vi "UHR-Fleezers Control (fpga) - 10.8b.vi"() -> ()   [LabVIEW 2014]
doc: "UHR-Fleezers Instrument Control Code (fpga)"
uses:
  <vilib>/eio/EIONode/EIONode.xnode
  <vilib>/eio/EIOMethodNode/EIOMethodNode.xnode
  <vilib>/rvi/DataTransferAndStorage/Container/XNode/niFpgaContainer.xnode
  <vilib>/Platform/TimedLoop/XDataNode/XDataNode.xnode
  <vilib>/Platform/TimedLoop/XDataNode/nitl_modes.ctl
  <vilib>/Platform/TimedLoop/XDataNode/XDNodeRunTimeDep.lvlib
  <vilib>/Platform/TimedLoop/XDataNode/wakeup.ctl
  <vilib>/Platform/TimedLoop/XDataNode/timing_clust.ctl
  <vilib>/addons/control/pid/fpga.llb/XNode/niFpgaPID.xnode
  <vilib>/rvi/eio/common/nirviEmuTemplateMethod_errors.vi
  <vilib>/rvi/interface/RandomDataEmulation/nirviRandomDataFpgaReadWriteTemplate.vi
panel:
  in  "Connector0/AO6":i16
  in  "Tab Control":T1(tab)=enum."Force FB"
  in  "Trap Pos to FIFO":bool
  in  "AI1 Sets to FIFO":T2={"Set 1"=TRUE, "Set 2"=TRUE, "Set 3"=FALSE}
  in  "N of AI1 Int Acq Sets":i16=2 min=1 max=3 step=1
  out "AI Late Counter":u16
  in  "ai count":u32=400
  out "AI late?":bool
  in  "+ phase":bool
  in  "Phase count adjustment":i16
  out "Relative phase":i16
  in  "AI to FIFO":bool
  out "BD1 Frequency Out 1":u64
  out "BD1 Frequency Out 2":u64
  out "Trap Pos FIFO Timeout":u16
  out "Trap AI FIFO Timeout":u16
  in  "Trap FIFO Set Timeout":i32
  in  "Tab Control 2":T3(tab)
  out "Wiggling 2":bool
  in  "Abort wiggle 2":bool
  in  "Wiggle amp 2":u64
  in  "Wiggle freq 2 (Hz)":fxp<+/-,16,16>
  in  "Wiggle trap 2":bool
  out "Wiggling 1":bool
  in  "Abort wiggle 1":bool
  in  "Wiggle trap 1":bool
  in  "Wiggle amp 1":u64
  in  "Wiggle freq 1 (Hz)":fxp<+/-,16,16>
  in  "Swap F1 and F2":bool
  in  "Freq or Amp switch first":bool=TRUE
  in  "Cont. Scan":bool
  in  "Abort scan":bool
  in  "Cycles per step":u64
  in  "Scan BD":bool
  in  "Number of scans":u16
  in  "Scan steps":u64
  in  "Scan freq.  increment":i64
  out "Scanning":bool
  in  "Start scan":bool
  in  "OSK Bd 1":bool
  in  "Reset Bd 1":bool
  in  "RD":bool
  in  "PMODE":bool
  in  "OSK Bd 2":bool
  in  "Reset Bd 2":bool
  in  "Direct RF Box \nCommunication":bool
  in  "Data BD 2":u8 format="%08b"
  in  "Data BD 1":u8 format="%08b"
  in  "Address":u8 format="%02x"
  in  "Update Data":bool
  in  "FPGA Controls\n RF Box":bool
  in  "Number Interlace Cycles":u8=2 min=1 max=3
  in  "Interlace Off Parameters":u8=1 min=1 max=3
  in  "Interlace ON/OFF":bool
  out "DIO Relative phase":i16
  in  "Phase count adjustment (DIO)":i16
  in  "+ phase (DIO)":bool
  out "DIO Late Counter":u16
  out "DIO Late?":bool
  in  "DIO count 1 (ticks)":u32=400
  in  "DIO count 2 (ticks)":u32=400
  in  "DIO count 3 (ticks)":u32=400
  out "AI2 Y Sum Set 2":i16
  out "AI2 Y Sum Set 1":i16
  in  "FB Gains Set 1":T4={"proportional gain (Kc)"=10, "integral gain (Kc*Ts/Ti)"=5, "derivative gain (Kc*Td/Ts)"=0}
  in  "FB Setpoint Set 1":i16 min=0 step=1
  in  "FB Reset Set 1":bool
  in  "FB On/Off Set 1":bool
  in  "FB Reset Set 2":bool
  in  "FB On/Off Set 2":bool
  in  "FB Setpoint Set 2":i16 min=0 step=1
  in  "FB Gains Set 2":T4={"proportional gain (Kc)"=10, "integral gain (Kc*Ts/Ti)"=5, "derivative gain (Kc*Td/Ts)"=0}
  in  "FB output range 2":cluster{"output high":i16, "output low":i16}={"output high"=3000, "output low"=0}
  in  "FB output range 1":cluster{"output high":i16, "output low":i16}={"output high"=3000, "output low"=0}
  out "Scan I":u64
  in  "Amp switch delay":u16=5
  in  "Freq switch delay":u16
  in  "BD 2 Amplitude 1":u16
  in  "BD 1 Amplitude 1":u16
  in  "BD 2 Frequency 1":u64
  in  "BD 1 Frequency 1":u64
  in  "BD 2 Amplitude 2":u16
  in  "BD 1 Amplitude 2":u16
  in  "BD 2 Frequency 2":u64
  in  "BD 1 Frequency 2":u64
  in  "BD 2 Amplitude 3":u16
  in  "BD 1 Amplitude 3":u16
  in  "BD 2 Frequency 3":u64
  in  "BD 1 Frequency 3":u64
  in  "Negate Diff?":bool
  in  "Diff FB Measurement?":bool
  in  "FB Trig Integrate":u32=1
  out "TTrig?":bool
  in  "TTrig Negate Pos":bool=TRUE
  out "Trap Pos FB Int Signal":fxp<+/-,24,9> format="%.18g"
  out "Trap Pos FB Int-Norm Signal":fxp<+/-,16,1> format="%.16g"
  in  "FPGA TTrig Thresh":i64
  in  "FPGA Trap Trig":bool
  out "Trap Pos FB Action":i64
  in  "Trap Pos. FB Offset Factor":i64
  in  "Trap Pos. FB Mult Factor":i64=2
  in  "Trap Pos. FB Range":T5={"output high"=0.999969482421875, "output low"=-1.0}
  in  "Trap Pos. FB Gains":T6={"proportional gain (Kc)"=0.0, "integral gain (Kc*Ts/Ti)"=10.0, "derivative gain (Kc*Td/Ts)"=0.0} {"proportional gain (Kc)" format="%.11g"; "integral gain (Kc*Ts/Ti)" format="%.11g"; "derivative gain (Kc*Td/Ts)" format="%.11g"}
  in  "Trap Pos. FB Reset":bool
  in  "Trap Pos FB Monitor T1 or T2":bool
  in  "AI1 X Scale":u16
  in  "Trap Pos FB Int Count":u16=100
  in  "Trap Pos FB Negate Action":bool
  out "AI1 X Set 2":fxp<+/-,16,1>
  out "AI1 X Set 1":fxp<+/-,16,1>
  in  "Trap Pos. FB SP":fxp<+/-,16,1>
  in  "Force feedback":bool
  out "TTrig Sig":i64
  out "TTrig Fin Thresh":i64
  out "Numeric":i32
  out "AO2 2":i16
  out "AO1 2":i16
  in  "1D or 2D Scan?":bool
  in  "Abort scan (MCL)":bool
  in  "MCL Scan Axis":bool
  in  "Cont. Scan (MCL)":bool
  out "Scan I (MCL)":u64
  in  "Number of scans (MCL)":u16
  out "Scanning MCL":bool
  in  "Scan steps (MCL)":u64
  in  "Cycles per step (MCL)":u64
  in  "Scan freq.  increment (MCL)":i16
  in  "Start scan (MCL)":bool
  in  "AO2":i16
  in  "AO1":i16
  out "MCL Late Counter":u16
  out "MCL Late?":bool
  in  "MCL count":u32=800
  out "MCL Relative Phase":i16
  in  "Phase count adjustment (MCL)":i16
  in  "+ phase (MCL)":bool
  in  "APD Gate Operating Mode":u8 max=2 step=1
  in  "Invert APD Gate":bool
  in  "APD Gate OFF Count":u32=100
  in  "APD Gate ON Count":u32=300
  out "APD 1 Gate Late Counter":u16
  out "APD 1 Gate Late?":bool
  out "APD 1 Gate Relative Phase":i16
  in  "Phase count adjustment (APD 1 Gate)":i16
  in  "+ phase (APD 1 Gate)":bool
  out "APD 2 Counts 0":u32
  out "APD 2 Counts 1":u32
  out "APD 1 Counts 0":u32
  out "APD 1 Counts 1":u32
  out "APD 1 out state":bool
  in  "APD 2 AO scale factor":i16=1
  in  "APD 1 AO scale factor":i16=1
  in  "APD to FIFO":bool
  in  "APD Acq Rate Count":u32=20000000
  out "APD Acq Late Counter":u16
  out "APD Acq Late?":bool
  out "APD Acq Relative Phase":i16
  in  "Phase Count Adjustment (APD Acq)":i16
  in  "+ phase (APD Acq)":bool
  in  "Phase count adjustment (APD 2 Gate)":i16
  out "APD 2 Gate Late Counter":u16
  out "APD 2 Gate Late?":bool
  out "APD 2 Gate Relative Phase":i16
  in  "+ phase (APD 2 Gate)":bool
  out "APD 2 out state":bool
  out "APD 1 Int Gate":bool
  out "APD 2 Int Gate":bool
  in  "Green Filter Flipper":bool
  out "Green FB Signals":T7
  in  "Green FB Count":u32=1200
  out "Green Late Counter":u16
  out "Green FB Late?":bool
  out "Green FB Relative Phase":i16
  in  "Phase count adjustment (Green FB)":i16=10
  in  "+ phase (Green FB)":bool
  out "Green FB Sum":i16
  in  "Green int current ON count adj":u32=150
  in  "Current Out":u16=30000
  in  "Green FB On/Off":bool
  in  "Green FB Setpoint":i16=250 min=0 step=1
  in  "Green FB Gains":T4={"proportional gain (Kc)"=10, "integral gain (Kc*Ts/Ti)"=5, "derivative gain (Kc*Td/Ts)"=0}
  in  "Green FB Reset":bool
  in  "Operating Mode 2":u8=2 max=2 step=1
  in  "Invert GI 2":bool
  in  "Green interlace OFF count 2":u32=900
  in  "Green interlace ON count 2":u32=300
  out "GI Late Counter 2":u16
  out "GI Late? 2":bool
  out "GI Relative phase 2":i16
  in  "Phase count adjustment (GI) 2":i16=20
  in  "+ phase (GI) 2":bool
  in  "Green interlace OFF count":u32=100
  out "GI Relative phase":i16
  in  "Phase count adjustment (GI)":i16
  in  "+ phase (GI)":bool
  in  "Green interlace ON count":u32=300
  out "GI Late Counter":u16
  in  "Invert GI":bool
  in  "Operating Mode":u8 max=2 step=1
  in  "RI Current Out":u16
  in  "RI operating mode 2":u8
  in  "Red operating mode":u8
  in  "Chassis2/Mod4/AO1":u16
  # "Only one of these can be on\nat a time:"
  # "Raster Scan AOD"
  # "1 (X)"
  # "2 (Y)"
  # "IR Intensity Feedback (RF BD 1)"
  # "FB Triggering Excitation Laser"
  # "AO1 (Y)"
  # "2D"
  # "1D"
  # "AO2 (X)"
  # "APD AO for aligning"
  # "Detection Loop"
  # "Green fluorescent laser digital gate interlacing loop"
  # "0 Forced ON\n1 Forced OFF\n2 Interlacing"
  # "Red fluorescent laser digital gate interlacing loop"
  # "0 Forced ON\n1 Forced OFF\n2 Interlacing"
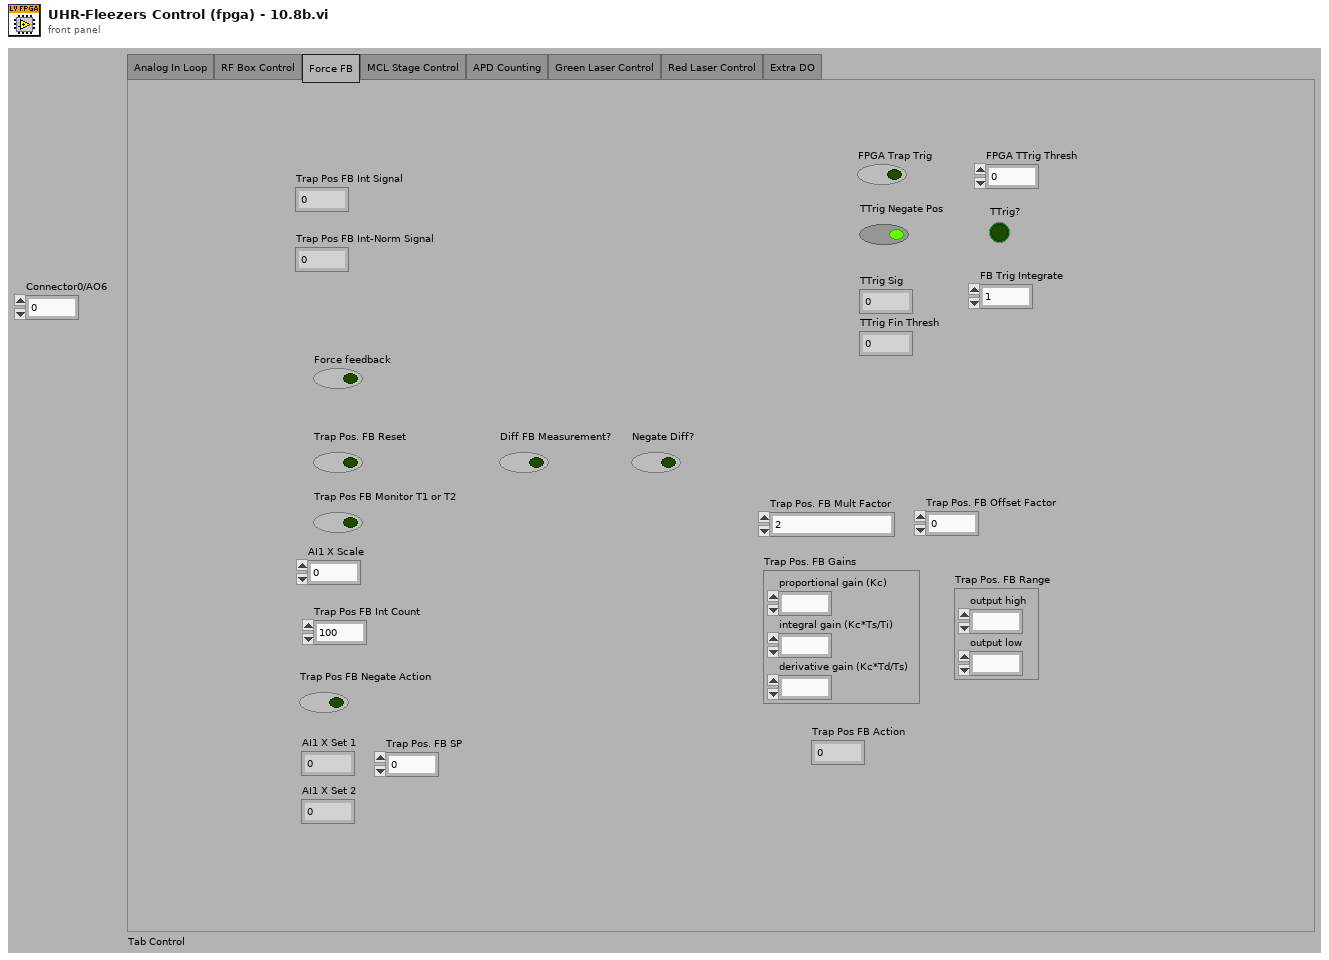
[diagram p1: front panel]
types:
  T1 = enum32{"Analog In Loop", "RF Box Control", "Force FB", "MCL Stage Control", "APD Counting", "Green Laser Control", "Red Laser Control", "Extra DO"}
  T2 = cluster{"Set 1":bool, "Set 2":bool, "Set 3":bool}
  T3 = enum32{"Controls", "Interlacing Frequency and Amplitude Values"}
  T4 = cluster{"proportional gain (Kc)":i16, "integral gain (Kc*Ts/Ti)":i16, "derivative gain (Kc*Td/Ts)":i16}
  T5 = cluster{"output high":fxp<+/-,16,1>, "output low":fxp<+/-,16,1>}
  T6 = cluster{"proportional gain (Kc)":fxp<+/-,16,8>, "integral gain (Kc*Ts/Ti)":fxp<+/-,16,8>, "derivative gain (Kc*Td/Ts)":fxp<+/-,16,8>}
  T7 = cluster{"Green FB Ch 0":i16, "Green FB Ch 1":i16, "Green FB Ch 2":i16}
  T8 = typedef "XDNodeRunTimeDep.lvlib/timing_clust.ctl" = cluster{"Expected End [f-1]":u64, "Actual End [f-1]":u64, "Finished Late? [f-1]":bool, "Expected End [i-1]":u64, "Actual End [i-1]":u64, "Finished Late? [i-1]":bool, "Expected Start [i]":u64, "Actual Start [i]":u64, "Expected Start [f]":u64, "Actual Start [f]":u64, "Source Name":string, "Structure Name":string, "Period":i64, "Deadline":i64, "Offset":i64, "Start":i64, "Priority":i32, "Timeout":i32, "Mode":T9, "Wakeup Reason":T10, "Error":errorcluster, "Source Type":string, "Secondary Source Type":string, "Global End Time":u64, "Global Start Time":u64, "Frame Duration":u64, "Iteration Duration":u64, "Assigned CPU":i32, "I/O Scan Engine Mode":u32}
  T9 = typedef "XDNodeRunTimeDep.lvlib/nitl_modes.ctl" = enum32{"No Change", "Process missed periods, maintain original phase", "Discard missed periods, maintain original phase", "Process missed periods, ignore original phase", "Discard missed periods, ignore original phase"}
  T10 = typedef "XDNodeRunTimeDep.lvlib/wakeup.ctl" = enum32{"Normal", "Aborted", "Asynchronous wakeup", "Timing source error", "Timed loop error", "Timeout"}
  T11 = cluster{"Chassis2/Mod1/AI0":void, "Chassis2/Mod1/AI1":void, "Chassis2/Mod1/AI2":void}
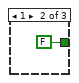
[diagram p2: hidden frame]
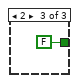
[diagram p3: hidden frame]
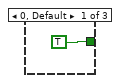
[diagram p4: hidden frame]
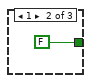
[diagram p5: hidden frame]
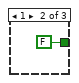
[diagram p6: hidden frame]
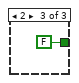
[diagram p7: hidden frame]
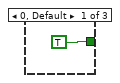
[diagram p9: hidden frame]
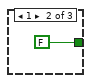
[diagram p10: hidden frame]
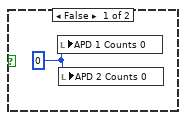
[diagram p11: hidden frame]
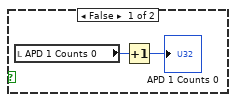
[diagram p14: hidden frame]
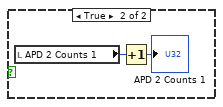
[diagram p16: hidden frame]
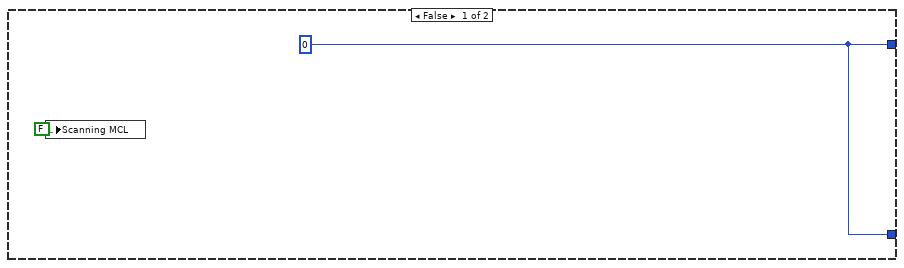
[diagram p17: hidden frame]
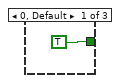
[diagram p18: hidden frame]
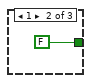
[diagram p19: hidden frame]
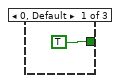
[diagram p20: hidden frame]
diagram:
  w1 = u16 0
  w4 = FALSE
  w2 = FALSE
  # "The APD Int Gate is here so the FPGA will do the integration only when the APD gate is \"ON\" (though we will leave the APD continuously ON now). This was added because the actual APD gating (via the hardware) was giving false signals. -KW"
  # "timing array current index"
  # "timing array"
  # "timing counter (phase adjusted here)"
  # "late counter"
  n1 = flat-sequence "FPGA initialization to do before running any of the loops" {
    tunnel: [u32 0 ("DIO count 3 (ticks)")] -> w3
    tunnel: [w10] -> _
    frame #0 {
      # "Start up expansion chassis early\nto avoid delays later"
      # "This pin controls udclk on the RF boards.\nWhen initially configuring the boards, this pin needs to be\nconfigured as a high impedance input.  Later it will be switched\nto an output."
      # "Initial setting of DIO data and \naddress to low (before reset).  \nThis needs to happen before the other\ncontrol method loops execute."
      n2 = xnode "FPGA I/O Node"("Chassis2/Mod4/AO0"=u16 0) -> ("Chassis2/Mod1/AI0"=w10)  [unwired: 2 in, 2 out]
      n3 = xnode "FPGA I/O Method Node"("Enable"=FALSE) -> ()  [unwired: 1 in, 1 out]
      n4 = xnode "FPGA I/O Node"("Connector1/DIO0"=FALSE, "Connector1/DIO1"=FALSE, "Connector1/DIO2"=FALSE, "Connector1/DIO3"=FALSE, "Connector1/DIO4"=FALSE, "Connector1/DIO5"=FALSE, "Connector1/DIO6"=FALSE, "Connector1/DIO7"=FALSE, "Connector1/DIO8"=FALSE, "Connector1/DIO9"=FALSE, "Connector1/DIO10"=FALSE, "Connector1/DIO11"=FALSE, "Connector1/DIO12"=FALSE, "Connector1/DIO13"=FALSE, "Connector1/DIO15"=FALSE, "Connector1/DIO20"=FALSE, "Connector1/DIO21"=FALSE, "Connector1/DIO22"=FALSE, "Connector1/DIO23"=FALSE, "Connector1/DIO24"=FALSE, "Connector1/DIO25"=FALSE, "Connector1/DIO26"=FALSE, "Connector1/DIO27"=FALSE, "Connector1/DIO14"=FALSE) -> ()  [unwired: 24 in, 24 out]
    }
  }
  n5 = local read "AO1"() -> (w8:i16)
  n6 = local read "AO2"() -> (w7:i16)
  n7 = node-c288() -> (w6:T8)  [unwired: 1 in]
  n8 = while "APD 1 Counter" {
    tunnel: w3 -> [_]
    stop <- FALSE stop-if-true
    n9 = flat-sequence {
      frame #0 {
        n10 = xnode "FPGA I/O Method Node"("FPGA I/O In"=refnum<k21> "Connector0/DIO0" ("APD 1 DO"), "Timeout"=-1) -> ()  [unwired: 2 out]
      }
      frame #1 {
        n11 = local read "APD 1 Int Gate"() -> (w41:bool)
        n12 = case shown="True" w41 {
          frame False {
          }
          frame True {
            n13 = local read "APD 1 out state"() -> (w42:bool)
            n14 = case shown="True" w42 {
              frame False {
                n15 = local read "APD 1 Counts 0"() -> (w44:u32)
                n16 = Increment(x=w44) -> (x+1=→"APD 1 Counts 0":u32)
              }
              frame True {
                n17 = local read "APD 1 Counts 1"() -> (w46:u32)
                n18 = Increment(x=w46) -> (x+1=→"APD 1 Counts 1":u32)
              }
            }
          }
        }
      }
    }
  }
  n19 = while "APD 2 Counter" {
    tunnel: w3 -> [_]
    stop <- FALSE stop-if-true
    n20 = flat-sequence {
      frame #0 {
        n21 = xnode "FPGA I/O Method Node"("FPGA I/O In"=refnum<k21> "Connector0/DIO1" ("APD 2 DO"), "Timeout"=-1) -> ()  [unwired: 2 out]
      }
      frame #1 {
        n22 = local read "APD 2 Int Gate"() -> (w50:bool)
        n23 = case shown="True" w50 {
          frame False {
          }
          frame True {
            n24 = local read "APD 2 out state"() -> (w51:bool)
            n25 = case shown="False" w51 {
              frame False {
                n26 = local read "APD 2 Counts 0"() -> (w53:u32)
                n27 = Increment(x=w53) -> (x+1=→"APD 2 Counts 0":u32)
              }
              frame True {
                n28 = local read "APD 2 Counts 1"() -> (w55:u32)
                n29 = Increment(x=w55) -> (x+1=→"APD 2 Counts 1":u32)
              }
            }
          }
        }
      }
    }
  }
  n30 = while "APD 2 Gating" {
    shift-right: [w59] -> _
    shift-left: w3 -> [w64]
    shift-right: [w58] -> _
    shift-left: w4 -> [w56]
    stop <- FALSE stop-if-true
    n31 = flat-sequence {
      tunnel: w64 -> [w67]
      tunnel: [w68] -> w62
      tunnel: [w67] -> w60
      tunnel: [w66] -> w57
      tunnel: w56 -> [w66]
      tunnel: [w71] -> w63
      tunnel: w62 -> [w71]
      tunnel: [w70] -> w61
      tunnel: w60 -> [w70]
      tunnel: w57 -> [w69]
      tunnel: [w89] -> w59
      tunnel: w63 -> [w100]
      tunnel: w61 -> [w98]
      tunnel: [w93] -> w58
      frame #0 {
        n32 = call "Loop Timer8"("Count(Ticks)"=w67) -> ("Tick Count(Ticks)"=w68:u32)
      }
      frame #1 {
        # "(need 4 channels/APD)"
        n33 = xnode "FPGA I/O Node"("Connector0/DIO8"=w69, "Connector0/DIO9"=w69, "Connector0/DIO10"=w69, "Connector0/DIO11"=w69) -> ()  [unwired: 4 in, 4 out]
        "APD 2 Int Gate" <- w69
      }
      frame #2 {
        n34 = local read "APD Gate ON Count"() -> (w82:u32)
        n35 = local read "APD Gate OFF Count"() -> (w81:u32)
        n36 = feedback #1(TRUE) -> (w95:bool)
        n37 = feedback-in #2(w100) -> ()
        n38 = feedback #2(w100) -> (w83:u32)
        n39 = Not(x=w95) -> (.not. x?=w92:bool)
        n40 = feedback-in #1(w92) -> ()
        n41 = Subtract(x=w100, y=w83) -> (x-y=w99:u32)
        n42 = Select(t=w82, s=w92, f=w81) -> (s? t:f=w97:u32)
        n43 = Subtract(x=w99, y=w98) -> (x-y=w74:u32)
        n44 = Subtract(x=w97, y=w74) -> (x-y=w88:u32)
        n45 = Number To Boolean Array(number=w74) -> (Boolean array=w73:bool[])
        n46 = Or Array Elements(Boolean array=w73) -> (logical OR=w72:bool)
        "APD 2 Gate Late?" <- w72
        n47 = Boolean To (0,1)(Boolean="+ phase (APD 2 Gate)") -> (0, 1=w86:i16)
        n48 = Multiply(x=w86, y="Phase count adjustment (APD 2 Gate)") -> (x*y=w84:i16)
        n49 = Boolean To (0,1)(Boolean=w72) -> (0, 1=w79:i16)
        n50 = Add(x=w88, y=w84) -> (x+y=w89:u32)
        n51 = To Unsigned Word Integer(number=w79) -> (unsigned 16bit integer=w76:u16)
        n52 = feedback #3(i16 0) -> (w91:i16)
        n53 = Subtract(x=w91, y=w84) -> (x-y=w90:i16)
        "APD 2 Gate Relative Phase" <- w90
        n54 = feedback-in #3(w90) -> ()
        n55 = feedback #4(u16 0) -> (w77:u16)
        n56 = Add(x=w76, y=w77) -> (x+y=w75:u16)
        "APD 2 Gate Late Counter" <- w75
        n57 = feedback-in #4(w75) -> ()
        n58 = local read "APD Gate Operating Mode"() -> (w80:u8)
        n59 = case shown="2" w80 {
          tunnel: [TRUE FALSE w106] -> w93
          tunnel: w95 -> [_ _ w104]
          frame 0, Default {
          }
          frame 1 {
          }
          frame 2 {
            n60 = local read "Invert APD Gate"() -> (w103:bool)
            n61 = Not(x=w104) -> (.not. x?=w105:bool)
            n62 = Select(t=w105, s=w103, f=w104) -> (s? t:f=w106:bool)
          }
        }
      }
    }
  }
  n63 = while "APD 1 Gating" {
    shift-right: [w110] -> _
    shift-left: w3 -> [w115]
    shift-right: [w109] -> _
    shift-left: w4 -> [w107]
    stop <- FALSE stop-if-true
    n64 = flat-sequence {
      tunnel: w115 -> [w118]
      tunnel: [w119] -> w113
      tunnel: [w118] -> w111
      tunnel: [w117] -> w108
      tunnel: w107 -> [w117]
      tunnel: [w122] -> w114
      tunnel: w113 -> [w122]
      tunnel: [w121] -> w112
      tunnel: w111 -> [w121]
      tunnel: w108 -> [w120]
      tunnel: [w136] -> w110
      tunnel: w114 -> [w151]
      tunnel: w112 -> [w148]
      tunnel: [w140] -> w109
      frame #0 {
        n65 = call "Loop Timer7"("Count(Ticks)"=w118) -> ("Tick Count(Ticks)"=w119:u32)
      }
      frame #1 {
        # "(need 4 channels/APD)"
        n66 = xnode "FPGA I/O Node"("Connector0/DIO4"=w120, "Connector0/DIO5"=w120, "Connector0/DIO6"=w120, "Connector0/DIO7"=w120) -> ()  [unwired: 4 in, 4 out]
        "APD 1 Int Gate" <- w120
      }
      frame #2 {
        n67 = feedback #5(TRUE) -> (w143:bool)
        n68 = feedback-in #6(w151) -> ()
        n69 = feedback #6(w151) -> (w150:u32)
        n70 = Not(x=w143) -> (.not. x?=w139:bool)
        n71 = feedback-in #5(w139) -> ()
        n72 = Subtract(x=w151, y=w150) -> (x-y=w149:u32)
        n73 = Select(t="APD Gate ON Count", s=w139, f="APD Gate OFF Count") -> (s? t:f=w145:u32)
        n74 = Subtract(x=w149, y=w148) -> (x-y=w124:u32)
        n75 = Subtract(x=w145, y=w124) -> (x-y=w135:u32)
        n76 = Number To Boolean Array(number=w124) -> (Boolean array=w125:bool[])
        n77 = Or Array Elements(Boolean array=w125) -> (logical OR=w123:bool)
        "APD 1 Gate Late?" <- w123
        n78 = Boolean To (0,1)(Boolean="+ phase (APD 1 Gate)") -> (0, 1=w133:i16)
        n79 = Boolean To (0,1)(Boolean=w123) -> (0, 1=w130:i16)
        n80 = Multiply(x=w133, y="Phase count adjustment (APD 1 Gate)") -> (x*y=w131:i16)
        n81 = To Unsigned Word Integer(number=w130) -> (unsigned 16bit integer=w127:u16)
        n82 = Add(x=w135, y=w131) -> (x+y=w136:u32)
        n83 = feedback #7(i16 0) -> (w138:i16)
        n84 = Subtract(x=w138, y=w131) -> (x-y=w137:i16)
        "APD 1 Gate Relative Phase" <- w137
        n85 = feedback-in #7(w137) -> ()
        n86 = feedback #8(u16 0) -> (w128:u16)
        n87 = Add(x=w127, y=w128) -> (x+y=w126:u16)
        "APD 1 Gate Late Counter" <- w126
        n88 = feedback-in #8(w126) -> ()
        n89 = case shown="2" "APD Gate Operating Mode" {
          tunnel: [TRUE FALSE w157] -> w140
          tunnel: w143 -> [_ _ w154]
          frame 0, Default {
          }
          frame 1 {
          }
          frame 2 {
            n90 = Not(x=w154) -> (.not. x?=w156:bool)
            n91 = Select(t=w156, s="Invert APD Gate", f=w154) -> (s? t:f=w157:bool)
          }
        }
      }
    }
  }
  n92 = timed-loop "RF box board DIO control: control bits" {
    timing: w6 -> [_]
    timing-out: [_] -> w5
    tunnel: [w158] -> _
    tunnel: w3 -> [w158]
    stop <- FALSE stop-if-true
    n93 = xnode "FPGA I/O Node"("Connector1/DIO16"="RD", "Connector1/DIO17"="PMODE", "Connector1/DIO18"="OSK Bd 1", "Connector1/DIO19"="Reset Bd 1", "Connector1/DIO28"="OSK Bd 2", "Connector1/DIO29"="Reset Bd 2") -> ()  [unwired: 6 in, 6 out]
  }
  n94 = while "Green fluorescent laser interlacing (DO to IA 532 nm AOM ME amp)." {
    shift-right: [w171] -> _
    shift-left: w3 -> [w176]
    shift-right: [w170] -> _
    shift-left: w2 -> [w168]
    stop <- FALSE stop-if-true
    n95 = flat-sequence {
      tunnel: w176 -> [w179]
      tunnel: [w180] -> w174
      tunnel: [w179] -> w172
      tunnel: [w178] -> w169
      tunnel: w168 -> [w178]
      tunnel: [w183] -> w175
      tunnel: w174 -> [w183]
      tunnel: [w182] -> w173
      tunnel: w172 -> [w182]
      tunnel: w169 -> [w181]
      tunnel: [w192] -> w171
      tunnel: w175 -> [w212]
      tunnel: w173 -> [w209]
      tunnel: [w201] -> w170
      frame #0 {
        n96 = call "Loop Timer4"("Count(Ticks)"=w179) -> ("Tick Count(Ticks)"=w180:u32)
      }
      frame #1 {
        n97 = xnode "FPGA I/O Node"("Connector1/DIO37"=w181, "Connector1/DIO38"=w181, "Connector1/DIO39"=w181) -> ()  [unwired: 3 in, 3 out]
      }
      frame #2 {
        n98 = feedback-in #9(w212) -> ()
        n99 = feedback #9(w212) -> (w211:u32)
        n100 = Subtract(x=w212, y=w211) -> (x-y=w210:u32)
        n101 = Subtract(x=w210, y=w209) -> (x-y=w185:u32)
        n102 = Number To Boolean Array(number=w185) -> (Boolean array=w186:bool[])
        n103 = Or Array Elements(Boolean array=w186) -> (logical OR=w184:bool)
        n104 = Boolean To (0,1)(Boolean="+ phase (GI)") -> (0, 1=w197:i16)
        n105 = Multiply(x=w197, y="Phase count adjustment (GI)") -> (x*y=w194:i16)
        n106 = Boolean To (0,1)(Boolean=w184) -> (0, 1=w191:i16)
        n107 = To Unsigned Word Integer(number=w191) -> (unsigned 16bit integer=w188:u16)
        n108 = feedback #10(i16 0) -> (w195:i16)
        n109 = feedback #11(u16 0) -> (w189:u16)
        n110 = Add(x=w188, y=w189) -> (x+y=w187:u16)
        "GI Late Counter" <- w187
        n111 = feedback-in #11(w187) -> ()
        n112 = Subtract(x=w195, y=w194) -> (x-y=w193:i16)
        "GI Relative phase" <- w193
        n113 = feedback-in #10(w193) -> ()
        n114 = feedback #12(TRUE) -> (w204:bool)
        n115 = case shown="1" "Operating Mode" {
          tunnel: [TRUE FALSE w218] -> w201
          tunnel: w204 -> [_ _ w215]
          frame 0, Default {
          }
          frame 1 {
          }
          frame 2 {
            n116 = Not(x=w215) -> (.not. x?=w217:bool)
            n117 = Select(t=w217, s="Invert GI", f=w215) -> (s? t:f=w218:bool)
          }
        }
        n118 = Not(x=w204) -> (.not. x?=w200:bool)
        n119 = Select(t="Green interlace ON count", s=w200, f="Green interlace OFF count") -> (s? t:f=w206:u32)
        n120 = Subtract(x=w206, y=w185) -> (x-y=w198:u32)
        n121 = Add(x=w198, y=w194) -> (x+y=w192:u32)
        n122 = feedback-in #12(w200) -> ()
      }
    }
  }
  n123 = while "Green fluorescent laser interlacing (Current to IA 532 nm AOM ME amp)." {
    shift-right: [w227] -> _
    shift-left: w3 -> [w230]
    shift-right: [w224] -> _
    shift-left: w1 -> [w222]
    shift-right: [w219] -> _
    shift-left: w1 -> [w221]
    stop <- FALSE stop-if-true
    n124 = flat-sequence {
      tunnel: w230 -> [w234]
      tunnel: [w235] -> w229
      tunnel: [w234] -> w228
      tunnel: [w233] -> w223
      tunnel: w222 -> [w233]
      tunnel: w221 -> [w232]
      tunnel: [w232] -> w220
      tunnel: [w239] -> w226
      tunnel: w229 -> [w239]
      tunnel: [w238] -> w225
      tunnel: w228 -> [w238]
      tunnel: w223 -> [w237]
      tunnel: w220 -> [w236]
      tunnel: [w254] -> w227
      tunnel: [w271] -> w224
      tunnel: w226 -> [w284]
      tunnel: w225 -> [w281]
      tunnel: [w240] -> w219
      frame #0 {
        n125 = call "Loop Timer10"("Count(Ticks)"=w234) -> ("Tick Count(Ticks)"=w235:u32)
      }
      frame #1 {
        n126 = xnode "FPGA I/O Node"("Chassis2/Mod4/AO0"=w237, "Chassis2/Mod4/AO1"=w236) -> ()  [unwired: 2 in, 2 out]
      }
      frame #2 {
        n127 = feedback #13(TRUE) -> (w276:bool)
        n128 = Subtract(x="Green interlace OFF count 2", y="Green int current ON count adj") -> (x-y=w263:u32)
        n129 = Not(x=w276) -> (.not. x?=w273:bool)
        n130 = feedback-in #13(w273) -> ()
        n131 = feedback-in #14(w284) -> ()
        n132 = feedback #14(w284) -> (w283:u32)
        n133 = Add(x="Green int current ON count adj", y="Green interlace ON count 2") -> (x+y=w264:u32)
        n134 = Subtract(x=w284, y=w283) -> (x-y=w282:u32)
        n135 = Select(t=w264, s=w273, f=w263) -> (s? t:f=w278:u32)
        n136 = Subtract(x=w282, y=w281) -> (x-y=w247:u32)
        n137 = case shown="0, Default" "RI operating mode 2" {
          tunnel: [TRUE FALSE FALSE] -> w244
          frame 0, Default {
          }
          frame 1 {
          }
          frame 2 {
          }
        }
        n138 = case shown="2" "Operating Mode 2" {
          tunnel: [TRUE FALSE w304] -> w265
          tunnel: w276 -> [_ _ w301]
          frame 0, Default {
          }
          frame 1 {
          }
          frame 2 {
            n139 = Not(x=w301) -> (.not. x?=w303:bool)
            n140 = Select(t=w303, s="Invert GI 2", f=w301) -> (s? t:f=w304:bool)
          }
        }
        n141 = Subtract(x=w278, y=w247) -> (x-y=w258:u32)
        n142 = Number To Boolean Array(number=w247) -> (Boolean array=w248:bool[])
        n143 = Boolean To (0,1)(Boolean="+ phase (GI) 2") -> (0, 1=w260:i16)
        n144 = Or Array Elements(Boolean array=w248) -> (logical OR=w246:bool)
        "GI Late? 2" <- w246
        n145 = Boolean To (0,1)(Boolean=w246) -> (0, 1=w253:i16)
        n146 = Multiply(x=w260, y="Phase count adjustment (GI) 2") -> (x*y=w256:i16)
        n147 = To Unsigned Word Integer(number=w253) -> (unsigned 16bit integer=w249:u16)
        n148 = Add(x=w258, y=w256) -> (x+y=w254:u32)
        n149 = feedback #15(u16 0) -> (w251:u16)
        n150 = Add(x=w249, y=w251) -> (x+y=w250:u16)
        "GI Late Counter 2" <- w250
        n151 = feedback-in #15(w250) -> ()
        n152 = feedback #16(i16 0) -> (w257:i16)
        n153 = Subtract(x=w257, y=w256) -> (x-y=w255:i16)
        "GI Relative phase 2" <- w255
        n154 = feedback-in #16(w255) -> ()
        n155 = And(x=w265, y="Green FB On/Off") -> (x .and. y?=w266:bool)
        n156 = case shown="True" w266 {
          tunnel: "Current Out" -> [w288 _]
          tunnel: [w288 w293] -> w270
          frame False {
          }
          frame True {
            n157 = local read "Green FB Sum"() -> (w289:i16)
            n158 = call "Slower PID.vi"("process variable"=w289, "reset?"="Green FB Reset", "setpoint"="Green FB Setpoint", "PID gains (x 2^8)"="Green FB Gains", "output range"=cluster{"output high":i16, "output low":i16} {"output high"=32767, "output low"=-32768} ("Green FB output range")) -> ("output"=w297:i16)  [unwired: 10 out]
            n159 = To Long Integer(number=w297) -> (32bit integer=w290:i32)
            n160 = Add(x=w290, y=32768) -> (x+y=w292:i32)
            n161 = To Unsigned Word Integer(number=w292) -> (unsigned 16bit integer=w293:u16)
          }
        }
        n162 = Boolean To (0,1)(Boolean=w244) -> (0, 1=w243:i16)
        n163 = Boolean To (0,1)(Boolean=w265) -> (0, 1=w272:i16)
        n164 = To Unsigned Word Integer(number=w272) -> (unsigned 16bit integer=w269:u16)
        n165 = To Unsigned Word Integer(number=w243) -> (unsigned 16bit integer=w242:u16)
        n166 = Multiply(x=w269, y=w270) -> (x*y=w271:u16)
        n167 = Multiply(x=w242, y="RI Current Out") -> (x*y=w240:u16)
      }
    }
  }
  n168 = while "Green excitation laser feedback measurement" {
    shift-right: [w305] -> _
    shift-left: w3 -> [w310]
    stop <- FALSE stop-if-true
    n169 = flat-sequence {
      tunnel: w310 -> [w312]
      tunnel: [w313] -> w308
      tunnel: [w312] -> w306
      tunnel: [w320] -> w309
      tunnel: w308 -> [w320]
      tunnel: [w319] -> w307
      tunnel: w306 -> [w319]
      tunnel: [w332] -> w305
      tunnel: w309 -> [w343]
      tunnel: w307 -> [w340]
      frame #0 {
        n170 = call "Loop Timer9"("Count(Ticks)"=w312) -> ("Tick Count(Ticks)"=w313:u32)
      }
      frame #1 {
        n171 = xnode "FPGA I/O Node"("Connector1/DIO35"=TRUE) -> ("Chassis2/Mod1/AI0"=w318, "Chassis2/Mod1/AI1"=w317, "Chassis2/Mod1/AI2"=w314)  [unwired: 4 in, 4 out]
        "Green FB Sum" <- w314
        n172 = Bundle("Chassis2/Mod1/AI0"=w318, "Chassis2/Mod1/AI1"=w317, "Chassis2/Mod1/AI2"=w314) -> (→"Green FB Signals":T11)  [unwired: 1 out]
      }
      frame #2 {
        n173 = feedback-in #17(w343) -> ()
        n174 = feedback #17(w343) -> (w342:u32)
        n175 = Subtract(x=w343, y=w342) -> (x-y=w341:u32)
        n176 = xnode "FPGA I/O Node"("Connector1/DIO35"=FALSE) -> ()  [unwired: 1 in, 1 out]
        n177 = Subtract(x=w341, y=w340) -> (x-y=w322:u32)
        n178 = Subtract(x="Green FB Count", y=w322) -> (x-y=w336:u32)
        n179 = Number To Boolean Array(number=w322) -> (Boolean array=w323:bool[])
        n180 = Or Array Elements(Boolean array=w323) -> (logical OR=w321:bool)
        "Green FB Late?" <- w321
        n181 = Boolean To (0,1)(Boolean="+ phase (Green FB)") -> (0, 1=w334:i16)
        n182 = Boolean To (0,1)(Boolean=w321) -> (0, 1=w328:i16)
        n183 = Multiply(x=w334, y="Phase count adjustment (Green FB)") -> (x*y=w329:i16)
        n184 = Add(x=w336, y=w329) -> (x+y=w332:u32)
        n185 = To Unsigned Word Integer(number=w328) -> (unsigned 16bit integer=w325:u16)
        n186 = feedback #18(i16 0) -> (w331:i16)
        n187 = Subtract(x=w331, y=w329) -> (x-y=w330:i16)
        "Green FB Relative Phase" <- w330
        n188 = feedback-in #18(w330) -> ()
        n189 = feedback #19(u16 0) -> (w326:u16)
        n190 = Add(x=w325, y=w326) -> (x+y=w324:u16)
        "Green Late Counter" <- w324
        n191 = feedback-in #19(w324) -> ()
      }
    }
  }
  n192 = while "Control Additional IO (Green laser flip mount)" {
    stop <- FALSE stop-if-true
    n193 = xnode "FPGA I/O Node"("Connector0/DIO3"="Green Filter Flipper", "Chassis2/Mod4/AO1"="Chassis2/Mod4/AO1", "Connector0/AO6"="Connector0/AO6") -> ()  [unwired: 3 in, 3 out]
    n194 = call "Loop Timer2"("Count(Ticks)"=u32 40000 ("Extra DO Counts")) -> ()  [unwired: 1 out]
  }
  n195 = while "DAQ AI set 1" {
    shift-right: [w349] -> _
    shift-left: w3 -> [w354]
    stop <- FALSE stop-if-true
    n196 = flat-sequence {
      tunnel: w354 -> [w364]
      tunnel: [w365] -> w352
      tunnel: [w364] -> w351
      tunnel: [w375] -> w362
      tunnel: [w374] -> w361
      tunnel: [w373] -> w360
      tunnel: [w372] -> w359
      tunnel: [w371] -> w358
      tunnel: [w370] -> w357
      tunnel: [w369] -> w356
      tunnel: [w368] -> w355
      tunnel: [w367] -> w353
      tunnel: w352 -> [w367]
      tunnel: w351 -> [w366]
      tunnel: [w366] -> w350
      tunnel: [w404] -> w349
      tunnel: w362 -> [w432]
      tunnel: w361 -> [w396]
      tunnel: w360 -> [w397]
      tunnel: w359 -> [w431]
      tunnel: w358 -> [w420]
      tunnel: w357 -> [w419]
      tunnel: w356 -> [w418]
      tunnel: w355 -> [w417]
      tunnel: w353 -> [w414]
      tunnel: w350 -> [w411]
      frame #0 {
        n197 = call "Loop Timer3"("Count(Ticks)"=w364) -> ("Tick Count(Ticks)"=w365:u32)
      }
      frame #1 {
        n198 = xnode "FPGA I/O Node"("Connector1/DIO31"=TRUE ("Connector1/DIO33")) -> ("Connector0/AI0"=w375, "Connector0/AI1"=w374, "Connector0/AI2"=w373, "Connector0/AI3"=w372, "Connector0/AI4"=w371, "Connector0/AI5"=w370, "Connector0/AI6"=w369, "Connector0/AI7"=w368)  [unwired: 9 in, 9 out]
      }
      frame #2 {
        w400 = FALSE ("AI to FIFO")
        # "Adjust phase after data acquired if button pressed"
        n199 = feedback #20(i16 1) -> (w424:i16)
        n200 = Increment(x=w424) -> (x+1=w430:i16)
        n201 = Scale By Power Of 2(n="AI1 X Scale", x=w396) -> (x*2^n=w394:dbl)
        n202 = Greater?(x=w430, y="N of AI1 Int Acq Sets") -> (0:w427:bool)
        n203 = Select(t=i16 1, s=w427, f=w430) -> (s? t:f=w429:i16)
        n204 = feedback-in #20(w429) -> ()
        n205 = Divide(x=w394, y=w397) -> (x/y=w393:fxp<+/-,16,1>)
        n206 = feedback #21(w400) -> (w398:bool)
        n207 = feedback #22(w400) -> (w416:bool)
        n208 = case shown="1, Default" w424 {
          tunnel: w397 -> [w454 w462 _]
          tunnel: "AI1 Sets to FIFO" -> [w458 w466 w472]
          tunnel: [w457 w465 w471] -> w421
          tunnel: ["AI to FIFO" w464 w470] -> w415
          tunnel: w416 -> [_ w464 w470]
          tunnel: ["Trap Pos to FIFO" w463 w469] -> w399
          tunnel: w398 -> [_ w463 w469]
          tunnel: w393 -> [w453 w461 _]
          tunnel: [w452 w459 FALSE] -> w380
          tunnel: [w451 w460 u64 0 ("BD1 Frequency Out 2")] -> w379
          frame 1, Default {
            n209 = Unbundle By Name(w458) -> ("Set 1"=w457:bool)
            n210 = local read "BD1 Frequency Out 1"() -> (w451:u64)
            n211 = Compound Arithmetic op=AND("Trap Pos to FIFO", w457, "AI to FIFO") -> (w452:bool)
            "AI2 Y Sum Set 1" <- w454
            "AI1 X Set 1" <- w453
          }
          frame 2 {
            n212 = Unbundle By Name(w466) -> ("Set 2"=w465:bool)
            n213 = local read "BD1 Frequency Out 2"() -> (w460:u64)
            n214 = Compound Arithmetic op=AND(w463, w465, w464) -> (w459:bool)
            "AI2 Y Sum Set 2" <- w462
            "AI1 X Set 2" <- w461
          }
          frame 3 {
            n215 = Unbundle By Name(w472) -> ("Set 3"=w471:bool)
          }
        }
        n216 = And(x=w421, y=w415) -> (x .and. y?=w423:bool)
        n217 = case shown="True" w423 {
          tunnel: w432 -> [_ w486]
          tunnel: w396 -> [_ w485]
          tunnel: w397 -> [_ w484]
          tunnel: w431 -> [_ w483]
          tunnel: w420 -> [_ w482]
          tunnel: w419 -> [_ w481]
          tunnel: w418 -> [_ w480]
          tunnel: w417 -> [_ w479]
          tunnel: 0 ("DMA buffer timeout") -> [_ w488]
          frame False {
          }
          frame True {
            n218 = Build Array(w486, w485, w484, w483, w482, w481, w480, w479) -> (w487:void[])
            n219 = for {
              tunnel: w487 -> [w490] mode=indexing
              tunnel: w488 -> [w491]
              tunnel: [w489] -> w477 mode=indexing
              n220 = xnode ("FIFO Write")("Element"=w490, "Timeout"=w491) -> ("Timed Out?"=w489:bool)  [unwired: 1 in, 1 out]
            }
            n221 = Or Array Elements(Boolean array=w477) -> (logical OR=w474:bool)
            n222 = Boolean To (0,1)(Boolean=w474) -> (0, 1=w476:i16)
            n223 = feedback #23(u16 0) -> (w475:u16)
            n224 = Add(x=w476, y=w475) -> (x+y=w473:u16)
            "Trap AI FIFO Timeout" <- w473
            n225 = feedback-in #23(w473) -> ()
          }
        }
        n226 = feedback-in #21(w399) -> ()
        n227 = feedback-in #22(w415) -> ()
        n228 = case shown="True" w380 {
          tunnel: w379 -> [_ w438]
          tunnel: [u8 0 w435] -> w378
          frame False {
          }
          frame True {
            n229 = Split Number(x=w438) -> (hi(x)=w439:u32, lo(x)=w440:u32)
            n230 = Split Number(x=w439) -> (lo(x)=w441:u16)  [unwired: 1 out]
            n231 = Split Number(x=w440) -> (hi(x)=w442:u16, lo(x)=w443:u16)
            n232 = Build Array "BD 1 nu Stack"(w441, w442, w443) -> (w437:u16[])
            n233 = for {
              tunnel: w437 -> [w450] mode=indexing
              shift-right: [w446] -> w435
              shift-left: u8 0 -> [w447]
              n234 = xnode ("FIFO Method Node")("Element"=w450, "Timeout"="Trap FIFO Set Timeout") -> ("Timed Out?"=w449:bool)  [unwired: 1 in, 1 out]
              n235 = Boolean To (0,1)(Boolean=w449) -> (0, 1=w448:i16)
              n236 = To Unsigned Byte Integer(number=w448) -> (unsigned 8bit integer=w445:u8)
              n237 = Add(x=w445, y=w447) -> (x+y=w446:u8)
            }
          }
        }
        n238 = To Unsigned Word Integer(number=w378) -> (unsigned 16bit integer=w377:u16)
        n239 = feedback #24(u16 0) -> (w391:u16)
        n240 = Add(x=w377, y=w391) -> (x+y=w390:u16)
        "Trap Pos FIFO Timeout" <- w390
        n241 = feedback-in #24(w390) -> ()
        n242 = feedback-in #25(w414) -> ()
        n243 = feedback #25(w414) -> (w413:u32)
        n244 = Subtract(x=w414, y=w413) -> (x-y=w412:u32)
        n245 = xnode "FPGA I/O Node"("Connector1/DIO31"=FALSE ("Connector1/DIO34")) -> ()  [unwired: 1 in, 1 out]
        n246 = Subtract(x=w412, y=w411) -> (x-y=w382:u32)
        n247 = Boolean To (0,1)(Boolean="+ phase") -> (0, 1=w407:i16)
        n248 = Multiply(x=w407, y="Phase count adjustment") -> (x*y=w401:i16)
        n249 = Subtract(x="ai count", y=w382) -> (x-y=w405:u32)
        n250 = Number To Boolean Array(number=w382) -> (Boolean array=w383:bool[])
        n251 = feedback #26(i16 0) -> (w403:i16)
        n252 = Add(x=w405, y=w401) -> (x+y=w404:u32)
        n253 = Subtract(x=w403, y=w401) -> (x-y=w402:i16)
        "Relative phase" <- w402
        n254 = feedback-in #26(w402) -> ()
        n255 = Or Array Elements(Boolean array=w383) -> (logical OR=w381:bool)
        "AI late?" <- w381
        n256 = Boolean To (0,1)(Boolean=w381) -> (0, 1=w388:i16)
        n257 = To Unsigned Word Integer(number=w388) -> (unsigned 16bit integer=w385:u16)
        n258 = feedback #27(u16 0) -> (w386:u16)
        n259 = Add(x=w385, y=w386) -> (x+y=w384:u16)
        "AI Late Counter" <- w384
        n260 = feedback-in #27(w384) -> ()
      }
    }
  }
  n261 = while "MCL stage control" {
    shift-right: [w507] -> _
    shift-left: w3 -> [w510]
    shift-right: [w500] -> _
    shift-left: w8 -> [w497]
    shift-right: [w499] -> _
    shift-left: w7 -> [w495]
    i -> [w494]
    stop <- FALSE stop-if-true
    n262 = flat-sequence {
      tunnel: w510 -> [w514]
      tunnel: [w515] -> w506
      tunnel: [w514] -> w504
      tunnel: [w513] -> w498
      tunnel: w497 -> [w513]
      tunnel: [w512] -> w496
      tunnel: w495 -> [w512]
      tunnel: w506 -> [w519]
      tunnel: [w519] -> w505
      tunnel: w504 -> [w518]
      tunnel: [w518] -> w503
      tunnel: w498 -> [w517]
      tunnel: w496 -> [w516]
      tunnel: [w517] -> w493
      tunnel: [w516] -> w492
      tunnel: w505 -> [w529]
      tunnel: w503 -> [w528]
      tunnel: [w529] -> w509
      tunnel: [w528] -> w508
      tunnel: [w527] -> w502
      tunnel: [w526] -> w501
      tunnel: w493 -> [w521]
      tunnel: w492 -> [w520]
      tunnel: [w601] -> w507
      tunnel: w509 -> [w608]
      tunnel: w508 -> [w605]
      tunnel: w502 -> [w603]
      tunnel: w501 -> [w602]
      tunnel: [w603] -> w500
      tunnel: [w602] -> w499
      frame #0 {
        n263 = call "Loop Timer5"("Count(Ticks)"=w514) -> ("Tick Count(Ticks)"=w515:u32)
      }
      frame #1 {
        n264 = xnode "FPGA I/O Node"("Connector0/AO1"=w517, "Connector0/AO2"=w516) -> ()  [unwired: 2 in, 2 out]
      }
      frame #2 {
        n265 = local read "Scanning MCL"() -> (w541:bool)
        n266 = Or(x=w541, y="Start scan (MCL)") -> (x .or. y?=w536:bool)
        n267 = Not(x="Abort scan (MCL)") -> (.not. x?=w534:bool)
        n268 = And(x=w534, y=w536) -> (x .and. y?=w533:bool)
        n269 = case "Raster scan" shown="True" w533 {
          tunnel: [w542 w585] -> w538
          tunnel: "Start scan (MCL)" -> [_ w570]
          tunnel: [w542 w546] -> w522
          frame False {
            w542 = i16 0
            n270 = local write "Scanning MCL"(FALSE ("scanning")) -> ()
          }
          frame True {
            w556 = i16 0
            w555 = u64 0
            # "scan incr."
            # "freq. incr. mult."
            # "count steps"
            # "count number of cycles"
            n271 = feedback #28(w555) -> (w582:u64)
            n272 = Select(t=w555, s=w570, f=w582) -> (s? t:f=w584:u64)
            n273 = Increment(x=w584) -> (x+1=w581:u64)
            n274 = Greater?(x="Cycles per step (MCL)", y=w581) -> (0:w565:bool)
            n275 = Select(t=w581, s=w565, f=w555) -> (s? t:f=w580:u64)
            n276 = feedback-in #28(w580) -> ()
            n277 = feedback #29(w555) -> (w579:u64)
            n278 = Select(t=w555, s=w570, f=w579) -> (s? t:f=w574:u64)
            n279 = Increment(x=w574) -> (x+1=w578:u64)
            n280 = Add(x="Scan steps (MCL)", y="Scan steps (MCL)") -> (x+y=w577:u64)
            n281 = Select(t=w574, s=w565, f=w578) -> (s? t:f=w560:u64)
            n282 = Greater?(x=w577, y=w560) -> (0:w559:bool)
            n283 = Select(t=w560, s=w559, f=w555) -> (s? t:f=w575:u64)
            n284 = feedback-in #29(w575) -> ()
            n285 = Equal?(x="Scan steps (MCL)", y=w560) -> (x = y?=w564:bool)
            n286 = Greater?(x="Scan steps (MCL)", y=w574) -> (0:w573:bool)
            n287 = feedback #30(w556) -> (w576:i16)
            n288 = Select(t=w556, s=w570, f=w576) -> (s? t:f=w562:i16)
            n289 = Increment(x=w562) -> (x+1=w572:i16)
            n290 = Decrement(x=w562) -> (x-1=w571:i16)
            n291 = Select(t=w572, s=w573, f=w571) -> (s? t:f=w563:i16)
            n292 = Select(t=w562, s=w564, f=w563) -> (s? t:f=w561:i16)
            n293 = Select(t=w562, s=w565, f=w561) -> (s? t:f=w557:i16)
            n294 = Select(t=w557, s=w559, f=w556) -> (s? t:f=w558:i16)
            n295 = feedback-in #30(w558) -> ()
            n296 = feedback #31(w555) -> (w569:u64)
            n297 = Select(t=w555, s=w570, f=w569) -> (s? t:f=w544:u64)
            n298 = Increment(x=w544) -> (x+1=w566:u64)
            n299 = Select(t=w544, s=w559, f=w566) -> (s? t:f=w545:u64)
            n300 = Greater?(x="Number of scans (MCL)", y=w545) -> (0:w552:bool)
            n301 = Multiply(x="Scan freq.  increment (MCL)", y=w562) -> (x*y=w585:i16)
            n302 = Select(t=TRUE, s="Cont. Scan (MCL)", f=w552) -> (s? t:f=w551:bool)
            "Scanning MCL" <- w551
            n303 = Select(t=w545, s=w551, f=w555) -> (s? t:f=w567:u64)
            n304 = feedback-in #31(w567) -> ()
            n305 = Increment(x=w545) -> (x+1=→"Scan I (MCL)":u64)
            n306 = To Word Integer(number=w544) -> (16bit integer=w547:i16)
            n307 = Multiply(x=w547, y="Scan freq.  increment (MCL)") -> (x*y=w546:i16)
          }
        }
        n308 = Select(t=w522, s="1D or 2D Scan?", f=i16 0) -> (s? t:f=w523:i16)
        n309 = Select(t=w523, s="MCL Scan Axis", f=w538) -> (s? t:f=w537:i16)
        n310 = Select(t=w538, s="MCL Scan Axis", f=w523) -> (s? t:f=w539:i16)
        n311 = Add(x=w537, y="AO2") -> (x+y=w526:i16)
        n312 = Add(x="AO1", y=w539) -> (x+y=w527:i16)
        "AO1 2" <- w521
        "AO2 2" <- w520
      }
      frame #3 {
        n313 = feedback-in #32(w608) -> ()
        n314 = feedback #32(w608) -> (w607:u32)
        n315 = Boolean To (0,1)(Boolean="+ phase (MCL)") -> (0, 1=w599:i16)
        n316 = Subtract(x=w608, y=w607) -> (x-y=w606:u32)
        n317 = Multiply(x=w599, y="Phase count adjustment (MCL)") -> (x*y=w595:i16)
        n318 = Subtract(x=w606, y=w605) -> (x-y=w587:u32)
        n319 = Subtract(x="MCL count", y=w587) -> (x-y=w597:u32)
        n320 = feedback #33(i16 0) -> (w596:i16)
        n321 = Subtract(x=w596, y=w595) -> (x-y=w594:i16)
        "MCL Relative Phase" <- w594
        n322 = feedback-in #33(w594) -> ()
        n323 = Number To Boolean Array(number=w587) -> (Boolean array=w588:bool[])
        n324 = Or Array Elements(Boolean array=w588) -> (logical OR=w586:bool)
        "MCL Late?" <- w586
        n325 = Boolean To (0,1)(Boolean=w586) -> (0, 1=w593:i16)
        n326 = Add(x=w597, y=w595) -> (x+y=w601:u32)
        n327 = To Unsigned Word Integer(number=w593) -> (unsigned 16bit integer=w590:u16)
        n328 = feedback #34(u16 0) -> (w591:u16)
        n329 = Add(x=w590, y=w591) -> (x+y=w589:u16)
        "MCL Late Counter" <- w589
        n330 = feedback-in #34(w589) -> ()
      }
    }
    "Numeric" <- w494
  }
  n331 = while "RF box board direct communication loop" {
    tunnel: w3 -> [_]
    stop <- FALSE stop-if-true
    n332 = case "Whether to use direct communication method (only use one method at a time)" shown="True" "Direct RF Box \nCommunication" {
      frame False {
      }
      frame True {
        n333 = case shown="True" "Update Data" {
          frame False {
          }
          frame True {
            n334 = flat-sequence {
              frame #0 {
                n335 = First Call?() -> (First Call?: T/F=w613:bool)
                n336 = case shown="True" w613 {
                  frame False {
                  }
                  frame True {
                    # "If first time data updated, be sure to set WR high\nbefore setting data and address bits."
                    n337 = flat-sequence {
                      frame #0 {
                        n338 = xnode "FPGA I/O Node"("Connector1/DIO15"=TRUE) -> ()  [unwired: 1 in, 1 out]
                      }
                      frame #1 {
                        n339 = call "Wait"("Count(Ticks)"=u8 40 ("DO Delay 3 (Ticks)")) -> ()  [unwired: 1 out]
                      }
                    }
                  }
                }
              }
              frame #1 {
                n340 = Number To Boolean Array(number="Address") -> (Boolean array=w662:bool[])
                n341 = Number To Boolean Array(number="Data BD 1") -> (Boolean array=w663:bool[])
                n342 = Number To Boolean Array(number="Data BD 2") -> (Boolean array=w632:bool[])
                n343 = Index Array(array=w663, index=7) -> (element=w647:bool)
                n344 = Index Array(array=w663, index=6) -> (element=w646:bool)
                n345 = Index Array(array=w663, index=5) -> (element=w645:bool)
                n346 = Index Array(array=w663, index=4) -> (element=w644:bool)
                n347 = Index Array(array=w663, index=3) -> (element=w643:bool)
                n348 = Index Array(array=w663, index=2) -> (element=w642:bool)
                n349 = Index Array(array=w663, index=1) -> (element=w641:bool)
                n350 = Index Array(array=w663, index=0) -> (element=w640:bool)
                n351 = Index Array(array=w662, index=5) -> (element=w639:bool)
                n352 = Index Array(array=w662, index=4) -> (element=w638:bool)
                n353 = Index Array(array=w662, index=3) -> (element=w637:bool)
                n354 = Index Array(array=w662, index=2) -> (element=w636:bool)
                n355 = Index Array(array=w662, index=1) -> (element=w635:bool)
                n356 = Index Array(array=w662, index=0) -> (element=w634:bool)
                n357 = Index Array(array=w632, index=7) -> (element=w623:bool)
                n358 = Index Array(array=w632, index=6) -> (element=w622:bool)
                n359 = Index Array(array=w632, index=5) -> (element=w621:bool)
                n360 = Index Array(array=w632, index=4) -> (element=w620:bool)
                n361 = Index Array(array=w632, index=3) -> (element=w619:bool)
                n362 = Index Array(array=w632, index=2) -> (element=w618:bool)
                n363 = Index Array(array=w632, index=1) -> (element=w617:bool)
                n364 = Index Array(array=w632, index=0) -> (element=w616:bool)
                n365 = xnode "FPGA I/O Node"("Connector1/DIO0"=w647, "Connector1/DIO1"=w646, "Connector1/DIO2"=w645, "Connector1/DIO3"=w644, "Connector1/DIO4"=w643, "Connector1/DIO5"=w642, "Connector1/DIO6"=w641, "Connector1/DIO7"=w640, "Connector1/DIO8"=w639, "Connector1/DIO9"=w638, "Connector1/DIO10"=w637, "Connector1/DIO11"=w636, "Connector1/DIO12"=w635, "Connector1/DIO13"=w634, "Connector1/DIO20"=w623, "Connector1/DIO21"=w622, "Connector1/DIO22"=w621, "Connector1/DIO23"=w620, "Connector1/DIO24"=w619, "Connector1/DIO25"=w618, "Connector1/DIO26"=w617, "Connector1/DIO27"=w616) -> ()  [unwired: 22 in, 22 out]
              }
              frame #2 {
                # "wait and then apply write signal"
                n366 = call "Wait2"("Count(Ticks)"=u8 40 ("DO Delay 1 (Ticks)")) -> ()  [unwired: 1 out]
              }
              frame #3 {
                # "sending bit low writes data to board buffer"
                n367 = xnode "FPGA I/O Node"("Connector1/DIO15"=FALSE) -> ()  [unwired: 1 in, 1 out]
              }
              frame #4 {
                # "wait then return write signal"
                n368 = call "Wait3"("Count(Ticks)"=u8 40 ("DO Delay 2 (Ticks)")) -> ()  [unwired: 1 out]
              }
              frame #5 {
                # "sending bit high makes ready to\nwrite more data"
                n369 = xnode "FPGA I/O Node"("Connector1/DIO15"=TRUE) -> ()  [unwired: 1 in, 1 out]
              }
            }
          }
        }
      }
    }
  }
  n370 = while "Control APD data integration - stream to host" {
    shift-right: [w672] -> _
    shift-left: w3 -> [w677]
    stop <- FALSE stop-if-true
    n371 = flat-sequence {
      tunnel: w677 -> [w679]
      tunnel: [w680] -> w675
      tunnel: [w679] -> w673
      tunnel: [w688] -> w676
      tunnel: w675 -> [w688]
      tunnel: [w687] -> w674
      tunnel: w673 -> [w687]
      tunnel: [w686] -> w671
      tunnel: [w685] -> w670
      tunnel: [w722] -> w672
      tunnel: w676 -> [w734]
      tunnel: w674 -> [w731]
      tunnel: w671 -> [w715]
      tunnel: w670 -> [w714]
      frame #0 {
        n372 = call "Loop Timer6"("Count(Ticks)"=w679) -> ("Tick Count(Ticks)"=w680:u32)
      }
      frame #1 {
        n373 = flat-sequence {
          tunnel: [w690] -> w684
          tunnel: w684 -> [w692]
          tunnel: [w694] -> w683
          tunnel: [w693] -> w682
          tunnel: [w692] -> w681
          tunnel: [w700] -> w685
          tunnel: [w701] -> w686
          tunnel: w683 -> [w701]
          tunnel: w682 -> [w700]
          tunnel: w681 -> [w699]
          frame #0 {
            # "use two separate variable so each APD won't\nhave to wait to read"
            n374 = feedback #35(FALSE) -> (w689:bool)
            "APD 1 out state" <- w689
            "APD 2 out state" <- w689
            n375 = Not(x=w689) -> (.not. x?=w690:bool)
            n376 = feedback-in #35(w690) -> ()
          }
          frame #1 {
            n377 = local read "APD 1 Counts 1"() -> (w698:u32)
            n378 = local read "APD 1 Counts 0"() -> (w697:u32)
            n379 = local read "APD 2 Counts 1"() -> (w696:u32)
            n380 = local read "APD 2 Counts 0"() -> (w695:u32)
            n381 = Select(t=w698, s=w692, f=w697) -> (s? t:f=w694:u32)
            n382 = Select(t=w696, s=w692, f=w695) -> (s? t:f=w693:u32)
          }
          frame #2 {
            n383 = case shown="True" w699 {
              frame False {
                w702 = u32 0 ("APD 1 Counts 0")
                n384 = local write "APD 1 Counts 0"(w702) -> ()
                n385 = local write "APD 2 Counts 0"(w702) -> ()
              }
              frame True {
                w703 = u32 0 ("APD 1 Counts 1")
                n386 = local write "APD 1 Counts 1"(w703) -> ()
                n387 = local write "APD 2 Counts 1"(w703) -> ()
              }
            }
          }
        }
      }
      frame #2 {
        n388 = feedback-in #36(w734) -> ()
        n389 = feedback #36(w734) -> (w733:u32)
        n390 = Subtract(x=w734, y=w733) -> (x-y=w732:u32)
        n391 = Subtract(x=w732, y=w731) -> (x-y=w707:u32)
        n392 = case shown="True" "APD to FIFO" {
          tunnel: w715 -> [_ w737]
          tunnel: w714 -> [_ w735]
          frame False {
          }
          frame True {
            n393 = flat-sequence {
              tunnel: 0 ("Timeout") -> [w739]
              tunnel: w737 -> [w740]
              tunnel: [w739] -> w736
              tunnel: w736 -> [w742]
              tunnel: w735 -> [w741]
              frame #0 {
                n394 = xnode ("FIFO Write")("Element"=w740, "Timeout"=w739) -> ()  [unwired: 1 in, 2 out]
              }
              frame #1 {
                n395 = xnode ("FIFO Write")("Element"=w741, "Timeout"=w742) -> ()  [unwired: 1 in, 2 out]
              }
            }
          }
        }
        n396 = Subtract(x="APD Acq Rate Count", y=w707) -> (x-y=w723:u32)
        n397 = Number To Boolean Array(number=w707) -> (Boolean array=w708:bool[])
        n398 = Or Array Elements(Boolean array=w708) -> (logical OR=w706:bool)
        "APD Acq Late?" <- w706
        n399 = Boolean To (0,1)(Boolean=w706) -> (0, 1=w713:i16)
        n400 = To Unsigned Word Integer(number=w713) -> (unsigned 16bit integer=w710:u16)
        n401 = Boolean To (0,1)(Boolean="+ phase (APD Acq)") -> (0, 1=w719:i16)
        n402 = feedback #37(u16 0) -> (w711:u16)
        n403 = Add(x=w710, y=w711) -> (x+y=w709:u16)
        "APD Acq Late Counter" <- w709
        n404 = feedback-in #37(w709) -> ()
        n405 = Multiply(x=w719, y="Phase Count Adjustment (APD Acq)") -> (x*y=w716:i16)
        n406 = Add(x=w723, y=w716) -> (x+y=w722:u32)
        n407 = feedback #38(i16 0) -> (w721:i16)
        n408 = Subtract(x=w721, y=w716) -> (x-y=w718:i16)
        "APD Acq Relative Phase" <- w718
        n409 = feedback-in #38(w718) -> ()
        n410 = To Word Integer(number=w715) -> (16bit integer=w724:i16)
        n411 = To Word Integer(number=w714) -> (16bit integer=w725:i16)
        n412 = Multiply(x="APD 1 AO scale factor", y=w724) -> (x*y=w705:i16)
        n413 = Multiply(x="APD 2 AO scale factor", y=w725) -> (x*y=w704:i16)
        n414 = xnode "FPGA I/O Node"("Connector0/AO5"=w705, "Connector0/AO7"=w704) -> ()  [unwired: 2 in, 2 out]
      }
    }
  }
  n415 = while "RF box board DIO control: parallel communication" {
    shift-right: [w749] -> _
    shift-left: w3 -> [w748]
    shift-right: [w747] -> _
    shift-left: FALSE ("Swap F1 and F2") -> [w746]
    stop <- FALSE stop-if-true
    n416 = flat-sequence {
      tunnel: w746 -> [w753]
      tunnel: w748 -> [w751]
      tunnel: [w753] -> w745
      tunnel: [w752] -> w744
      tunnel: [w751] -> w743
      tunnel: [w759] -> w749
      tunnel: [w758] -> w747
      tunnel: w745 -> [w757]
      tunnel: w744 -> [w755]
      tunnel: w743 -> [w754]
      frame #0 {
        n417 = call "Loop Timer"("Count(Ticks)"=w751) -> ("Tick Count(Ticks)"=w752:u32)
      }
      frame #1 {
        n418 = flat-sequence {
          tunnel: ["FPGA Controls\n RF Box"] -> w756
          tunnel: w757 -> [w760]
          tunnel: [w800] -> w759
          tunnel: [w813] -> w758
          tunnel: w756 -> [w812]
          tunnel: w755 -> [w806]
          tunnel: w754 -> [w803]
          frame #0 {
            n419 = case shown="True" "FPGA Controls\n RF Box" {
              tunnel: w760 -> [_ w762]
              frame False {
              }
              frame True {
                n420 = flat-sequence {
                  tunnel: w762 -> [w768]
                  frame #0 {
                    n421 = First Call?() -> (First Call?: T/F=w763:bool)
                    n422 = case shown="True" w763 {
                      frame False {
                      }
                      frame True {
                        # "If first time data updated, be sure to set WR high and UDCLK low\nbefore setting data and address bits."
                        n423 = xnode "FPGA I/O Method Node"("Enable"=TRUE) -> ("FPGA I/O Out"=w765:refnum<k21>)  [unwired: 1 in]
                        n424 = xnode "FPGA I/O Node"("Connector1/DIO15"=TRUE) -> ()  [unwired: 1 in, 1 out]
                        n425 = xnode "FPGA I/O Node"("I/O Item"=FALSE ("Connector1/DIO30"), "FPGA I/O In"=w765) -> ()  [unwired: 1 out]
                      }
                    }
                  }
                  frame #1 {
                    n426 = case shown="True" "Freq or Amp switch first" {
                      tunnel: w768 -> [w770 w775]
                      frame False {
                        n427 = flat-sequence {
                          tunnel: w770 -> [w774]
                          frame #0 {
                            # "switch amplitude"
                            # "send udclk high"
                            n428 = xnode "FPGA I/O Node"("Connector1/DIO30"=TRUE ("Connector1/DIO15")) -> ()  [unwired: 1 in, 1 out]
                          }
                          frame #1 {
                            # "send udclk low"
                            n429 = xnode "FPGA I/O Node"("Connector1/DIO30"=FALSE ("Connector1/DIO15")) -> ()  [unwired: 1 in, 1 out]
                          }
                          frame #2 {
                            n430 = call "Wait5"("Count(Ticks)"="Freq switch delay") -> ()  [unwired: 1 out]
                          }
                          frame #3 {
                            # "switch frequency"
                            n431 = xnode "FPGA I/O Node"("Connector1/DIO36"=w774) -> ()  [unwired: 1 in, 1 out]
                          }
                        }
                      }
                      frame True {
                        n432 = flat-sequence {
                          tunnel: w775 -> [w776]
                          frame #0 {
                            # "switch frequency"
                            n433 = xnode "FPGA I/O Node"("Connector1/DIO36"=w776) -> ()  [unwired: 1 in, 1 out]
                          }
                          frame #1 {
                            n434 = call "Wait4"("Count(Ticks)"="Amp switch delay") -> ()  [unwired: 1 out]
                          }
                          frame #2 {
                            # "switch amplitude"
                            # "send udclk high"
                            n435 = xnode "FPGA I/O Node"("Connector1/DIO30"=TRUE ("Connector1/DIO15")) -> ()  [unwired: 1 in, 1 out]
                          }
                          frame #3 {
                            # "send udclk low"
                            n436 = xnode "FPGA I/O Node"("Connector1/DIO30"=FALSE ("Connector1/DIO15")) -> ()  [unwired: 1 in, 1 out]
                          }
                        }
                      }
                    }
                  }
                }
              }
            }
          }
          frame #1 {
            # "This is the prior cycle's on time"
            # "increment timing\nindex, reset to 0 if \nend of matrix"
            # "Reset to begginning (1) when number of cycles reached."
            # "timing index"
            # "build byte stacks for writing data\n(must correspond to addresses array constant)"
            # "Timing housekeeping"
            # "Adjust phase if late\n(maintains constant phase relationship between cycles)"
            n437 = feedback #39(u8 0 ("t")) -> (w809:u8)
            n438 = Increment(x=w809) -> (x+1=w853:u8)
            n439 = Increment(x="Number Interlace Cycles") -> (x+1=w848:u8)
            n440 = Equal?(x=w853, y=w848) -> (x = y?=w855:bool)
            n441 = Select(t=u8 1, s=w855, f=w853) -> (s? t:f=w808:u8)
            n442 = feedback-in #39(w808) -> ()
            n443 = Increment(x=w808) -> (x+1=w850:u8)
            n444 = Equal?(x=w850, y=w848) -> (x = y?=w851:bool)
            n445 = Select(t=u8 1, s=w851, f=w850) -> (s? t:f=w847:u8)
            n446 = Select(t=w847, s="Interlace ON/OFF", f="Interlace Off Parameters") -> (s? t:f=w831:u8)
            n447 = case shown="2" w831 {
              tunnel: [w925 w1090 "BD 1 Frequency 3"] -> w843
              tunnel: [w924 "BD 2 Frequency 2" "BD 2 Frequency 3"] -> w832
              tunnel: ["BD 2 Amplitude 1" "BD 2 Amplitude 2" "BD 2 Amplitude 3"] -> w788
              tunnel: [w914 w1100 "BD 1 Amplitude 3"] -> w791
              frame 1, Default {
                w905 = fxp<+/-,24,9> 0.0 ("AI1 X Set 2")
                w898 = u16 0
                w920 = u64 0 ("f")
                # "This signal integration happens no matter what\nso that correct setpoints can be chosen before \nturning on the FB."
                # "Trap 1"
                n448 = local read "AI1 X Set 2"() -> (w901:fxp<+/-,16,1>)
                n449 = local read "AI1 X Set 1"() -> (w902:fxp<+/-,16,1>)
                n450 = local read "Scanning"() -> (w926:bool)
                n451 = case shown="False" "Diff FB Measurement?" {
                  tunnel: w901 -> [w934 w943]
                  tunnel: w902 -> [w933 w944]
                  tunnel: [w931 w935] -> w903
                  frame False {
                    n452 = Select(t=w933, s="Trap Pos FB Monitor T1 or T2", f=w934) -> (s? t:f=w931:fxp<+/-,16,1>)
                  }
                  frame True {
                    n453 = Subtract(x=w944, y=w943) -> (x-y=w936:fxp<+/-,17,2>)
                    n454 = Not(x="Negate Diff?") -> (.not. x?=w942:bool)
                    n455 = Boolean To (0,1)(Boolean="Negate Diff?") -> (0, 1=w940:i16)
                    n456 = Boolean To (0,1)(Boolean=w942) -> (0, 1=w941:i16)
                    n457 = Negate(x=w940) -> (-x=w939:i16)
                    n458 = Add(x=w939, y=w941) -> (x+y=w937:i16)
                    n459 = Multiply(x=w937, y=w936) -> (x*y=w935:fxp<+/-,32,17>)
                  }
                }
                n460 = Or(x=w926, y="Start scan") -> (x .or. y?=w918:bool)
                n461 = Not(x="Abort scan") -> (.not. x?=w916:bool)
                n462 = And(x=w916, y=w918) -> (x .and. y?=w889:bool)
                n463 = feedback #40(w898) -> (w897:u16)
                n464 = Increment(x=w897) -> (x+1=w899:u16)
                n465 = Greater Or Equal?(x=w899, y="Trap Pos FB Int Count") -> (x >= y?=w890:bool)
                n466 = case "For raster scanning" shown="False" w889 {
                  tunnel: [w1031 w1043] -> w921
                  tunnel: "Start scan" -> [_ w1067]
                  frame False {
                    # "For wiggle-calibration: sinusoidal wave"
                    n467 = local read "Wiggling 1"() -> (w1026:bool)
                    n468 = Not(x="Abort wiggle 1") -> (.not. x?=w1029:bool)
                    n469 = Or(x="Wiggle trap 1", y=w1026) -> (x .or. y?=w1025:bool)
                    n470 = And(x=w1025, y=w1029) -> (x .and. y?=w1028:bool)
                    n471 = case shown="True" w1028 {
                      tunnel: [u64 0 w1039] -> w1031
                      frame False {
                        n472 = local write "Wiggling 1"(FALSE ("Wiggle")) -> ()
                      }
                      frame True {
                        # "Input is periods/tick, not Hz,\nso need to normalize by clock\nfrequency (40 MHz)."
                        n473 = Divide(x="Wiggle freq 1 (Hz)", y=fxp<+,17,26> 40000000.0) -> (x/y=w1036:fxp<+/-,17,-9>)
                        n474 = call "Sine Wave Generator"("frequency (periods/tick)"=w1036) -> ("sine out"=w1041:i32)  [unwired: 14 in]
                        n475 = Multiply(x=w1041, y="Wiggle amp 1") -> (x*y=w1039:u64)
                        "Wiggling 1" <- TRUE
                      }
                    }
                    n476 = local write "Scanning"(FALSE ("scanning")) -> ()
                  }
                  frame True {
                    w1051 = i64 0
                    w1050 = u64 0
                    # "scan incr."
                    # "freq. incr. mult."
                    # "count steps"
                    # "count number of cycles"
                    n477 = feedback #41(w1050) -> (w1079:u64)
                    n478 = Select(t=w1050, s=w1067, f=w1079) -> (s? t:f=w1081:u64)
                    n479 = Increment(x=w1081) -> (x+1=w1078:u64)
                    n480 = Greater?(x="Cycles per step", y=w1078) -> (0:w1060:bool)
                    n481 = Select(t=w1078, s=w1060, f=w1050) -> (s? t:f=w1077:u64)
                    n482 = feedback-in #41(w1077) -> ()
                    n483 = feedback #42(w1050) -> (w1076:u64)
                    n484 = Select(t=w1050, s=w1067, f=w1076) -> (s? t:f=w1071:u64)
                    n485 = Increment(x=w1071) -> (x+1=w1075:u64)
                    n486 = Add(x="Scan steps", y="Scan steps") -> (x+y=w1074:u64)
                    n487 = Select(t=w1071, s=w1060, f=w1075) -> (s? t:f=w1055:u64)
                    n488 = Greater?(x=w1074, y=w1055) -> (0:w1054:bool)
                    n489 = Select(t=w1055, s=w1054, f=w1050) -> (s? t:f=w1072:u64)
                    n490 = feedback-in #42(w1072) -> ()
                    n491 = Equal?(x="Scan steps", y=w1055) -> (x = y?=w1059:bool)
                    n492 = Greater?(x="Scan steps", y=w1071) -> (0:w1070:bool)
                    n493 = feedback #43(w1051) -> (w1073:i64)
                    n494 = Select(t=w1051, s=w1067, f=w1073) -> (s? t:f=w1057:i64)
                    n495 = Increment(x=w1057) -> (x+1=w1069:i64)
                    n496 = Decrement(x=w1057) -> (x-1=w1068:i64)
                    n497 = Select(t=w1069, s=w1070, f=w1068) -> (s? t:f=w1058:i64)
                    n498 = Select(t=w1057, s=w1059, f=w1058) -> (s? t:f=w1056:i64)
                    n499 = Select(t=w1057, s=w1060, f=w1056) -> (s? t:f=w1052:i64)
                    n500 = Select(t=w1052, s=w1054, f=w1051) -> (s? t:f=w1053:i64)
                    n501 = feedback-in #43(w1053) -> ()
                    n502 = feedback #44(w1050) -> (w1066:u64)
                    n503 = Select(t=w1050, s=w1067, f=w1066) -> (s? t:f=w1062:u64)
                    n504 = Increment(x=w1062) -> (x+1=w1063:u64)
                    n505 = Select(t=w1062, s=w1054, f=w1063) -> (s? t:f=w1061:u64)
                    n506 = Greater?(x="Number of scans", y=w1061) -> (0:w1047:bool)
                    n507 = Multiply(x="Scan freq.  increment", y=w1057) -> (x*y=w1043:i64)
                    n508 = Select(t=TRUE, s="Cont. Scan", f=w1047) -> (s? t:f=w1046:bool)
                    "Scanning" <- w1046
                    n509 = Select(t=w1061, s=w1046, f=w1050) -> (s? t:f=w1064:u64)
                    n510 = feedback-in #44(w1064) -> ()
                    n511 = Increment(x=w1061) -> (x+1=→"Scan I":u64)
                  }
                }
                n512 = Select(t=w898, s=w890, f=w899) -> (s? t:f=w900:u16)
                n513 = feedback-in #40(w900) -> ()
                n514 = feedback #45(w905) -> (w904:fxp<+/-,24,9>)
                n515 = Add(x=w903, y=w904) -> (x+y=w896:fxp<+/-,24,9>)
                n516 = Select(t=w905, s=w890, f=w896) -> (s? t:f=w908:fxp<+/-,24,9>)
                n517 = feedback-in #45(w908) -> ()
                n518 = Divide(x=w896, y="Trap Pos FB Int Count") -> (x/y=w891:fxp<+/-,16,1>)
                n519 = feedback #46(fxp<+/-,24,9> 0.0 ("AI1 X Set 2")) -> (w909:fxp<+/-,24,9>)
                n520 = Select(t=w896, s=w890, f=w909) -> (s? t:f=w910:fxp<+/-,24,9>)
                "Trap Pos FB Int Signal" <- w910
                n521 = feedback-in #46(w910) -> ()
                n522 = feedback #47(fxp<+/-,16,1> 0.0 ("Trap Pos FB Int-Norm Signal")) -> (w893:fxp<+/-,16,1>)
                n523 = Select(t=w891, s=w890, f=w893) -> (s? t:f=w892:fxp<+/-,16,1>)
                "Trap Pos FB Int-Norm Signal" <- w892
                n524 = feedback-in #47(w892) -> ()
                n525 = case "For position feedback" shown="True" "Force feedback" {
                  tunnel: [i64 0 w950] -> w911
                  tunnel: w891 -> [_ w947]
                  tunnel: w890 -> [_ w946]
                  frame False {
                  }
                  frame True {
                    n526 = feedback #48(i64 0) -> (w949:i64)
                    n527 = case shown="True" w946 {
                      tunnel: [w951 w958] -> w950
                      tunnel: w949 -> [w951 _]
                      tunnel: w947 -> [_ w952]
                      frame False {
                      }
                      frame True {
                        w962 = u32 0
                        n528 = xnode ("PID")("process variable"=w952, "reset?"="Trap Pos. FB Reset", "setpoint"="Trap Pos. FB SP", "PID gains"="Trap Pos. FB Gains", "output range"="Trap Pos. FB Range") -> ("output"=w974:fxp<+/-,16,1>)
                        n529 = Negate(x=w974) -> (-x=w973:fxp<+/-,17,2>)
                        n530 = Select(t=w973, s="Trap Pos FB Negate Action", f=w974) -> (s? t:f=w970:fxp<+/-,17,2>)
                        n531 = Scale By Power Of 2(n=u32 15, x=u32 1) -> (x*2^n=w967:u32)
                        n532 = Multiply(x=w970, y=w967) -> (x*y=w966:fxp<+/-,17,17>)
                        n533 = To Quad Integer(1:w966) -> (0:w978:i64)
                        "Trap Pos FB Action" <- w978
                        n534 = Multiply(x=w978, y="Trap Pos. FB Mult Factor") -> (x*y=w976:i64)
                        n535 = Add(x=w976, y="Trap Pos. FB Offset Factor") -> (x+y=w958:i64)
                        n536 = feedback #49() -> (w959:i64)  [unwired: 1 in]
                        n537 = Add(x=w958, y=w959) -> (x+y=w956:i64)
                        n538 = feedback #50(w962) -> (w964:u32)
                        n539 = Increment(x=w964) -> (x+1=w953:u32)
                        n540 = Greater Or Equal?(x=w953, y="FB Trig Integrate") -> (x >= y?=w954:bool)
                        n541 = Select(t=i64 0, s=w954, f=w956) -> (s? t:f=w960:i64)
                        n542 = feedback-in #49(w960) -> ()
                        n543 = Select(t=w962, s=w954, f=w953) -> (s? t:f=w963:u32)
                        n544 = feedback-in #50(w963) -> ()
                        n545 = And(x=w954, y="FPGA Trap Trig") -> (x .and. y?=w961:bool)
                        n546 = case "Trap FB trigger excitation laser ON" shown="True" w961 {
                          tunnel: w956 -> [_ w984]
                          tunnel: w953 -> [_ w982]
                          frame False {
                          }
                          frame True {
                            n547 = Not(x="TTrig Negate Pos") -> (.not. x?=w991:bool)
                            n548 = Boolean To (0,1)(Boolean="TTrig Negate Pos") -> (0, 1=w989:i16)
                            n549 = Boolean To (0,1)(Boolean=w991) -> (0, 1=w990:i16)
                            n550 = Negate(x=w989) -> (-x=w988:i16)
                            n551 = Add(x=w988, y=w990) -> (x+y=w987:i16)
                            n552 = Multiply(x=w987, y=w984) -> (x*y=w986:i64)
                            "TTrig Sig" <- w986
                            n553 = Multiply(x="FPGA TTrig Thresh", y=w982) -> (x*y=w983:i64)
                            "TTrig Fin Thresh" <- w983
                            n554 = Greater Or Equal?(x=w986, y=w983) -> (x >= y?=w985:bool)
                            n555 = case shown="True" w985 {
                              frame False {
                              }
                              frame True {
                                w994 = TRUE ("Green FB On/Off")
                                w996 = u8 2 ("Operating Mode")
                                n556 = local write "Operating Mode 2"(w996) -> ()
                                n557 = local write "Operating Mode"(w996) -> ()
                                n558 = local write "Green FB On/Off"(w994) -> ()
                                n559 = local write "FPGA Trap Trig"(FALSE ("FPGA Trap Trig")) -> ()
                                "TTrig?" <- w994
                              }
                            }
                          }
                        }
                      }
                    }
                    n560 = feedback-in #48(w950) -> ()
                  }
                }
                n561 = case "For intensity feedback" shown="True" "FB On/Off Set 1" {
                  tunnel: "BD 1 Amplitude 1" -> [w1082 _]
                  tunnel: [w1082 w1083] -> w914
                  frame False {
                  }
                  frame True {
                    n562 = local read "AI2 Y Sum Set 1"() -> (w1085:i16)
                    n563 = call "Slower PID.vi"("process variable"=w1085, "reset?"="FB Reset Set 1", "setpoint"="FB Setpoint Set 1", "PID gains (x 2^8)"="FB Gains Set 1", "output range"="FB output range 1") -> ("output"=w1088:i16)  [unwired: 10 out]
                    n564 = To Unsigned Word Integer(number=w1088) -> (unsigned 16bit integer=w1083:u16)
                  }
                }
                n565 = Select(t=w920, s="Scan BD", f=w921) -> (s? t:f=w919:u64)
                n566 = Select(t=w921, s="Scan BD", f=w920) -> (s? t:f=w922:u64)
                n567 = Add(x=w919, y="BD 2 Frequency 1") -> (x+y=w924:u64)
                n568 = Compound Arithmetic op=ADD("BD 1 Frequency 1", w911, w922) -> (w925:u64)
                "BD1 Frequency Out 1" <- w925
              }
              frame 2 {
                # "For wiggle calibration"
                # "Trap 2"
                n569 = local read "Wiggling 2"() -> (w1097:bool)
                n570 = Or(x="Wiggle trap 2", y=w1097) -> (x .or. y?=w1096:bool)
                n571 = Not(x="Abort wiggle 2") -> (.not. x?=w1094:bool)
                n572 = And(x=w1096, y=w1094) -> (x .and. y?=w1093:bool)
                n573 = case shown="True" "FB On/Off Set 2" {
                  tunnel: [w1113 w1114] -> w1100
                  tunnel: "BD 1 Amplitude 2" -> [w1113 _]
                  frame False {
                  }
                  frame True {
                    n574 = local read "AI2 Y Sum Set 2"() -> (w1119:i16)
                    n575 = call "Slower PID.vi"("process variable"=w1119, "reset?"="FB Reset Set 2", "setpoint"="FB Setpoint Set 2", "PID gains (x 2^8)"="FB Gains Set 2", "output range"="FB output range 2") -> ("output"=w1116:i16)  [unwired: 10 out]
                    n576 = To Unsigned Word Integer(number=w1116) -> (unsigned 16bit integer=w1114:u16)
                  }
                }
                n577 = case shown="True" w1093 {
                  tunnel: [i16 0 w1107] -> w1091
                  frame False {
                    n578 = local write "Wiggling 2"(FALSE) -> ()
                  }
                  frame True {
                    n579 = Divide(x="Wiggle freq 2 (Hz)", y=fxp<+,17,26> 40000000.0) -> (x/y=w1110:fxp<+/-,17,-9>)
                    n580 = call "Sine Wave Generator2"("frequency (periods/tick)"=w1110) -> ("sine out"=w1109:i32)  [unwired: 14 in]
                    n581 = Multiply(x=w1109, y="Wiggle amp 2") -> (x*y=w1107:u64)
                    "Wiggling 2" <- TRUE
                  }
                }
                n582 = Add(x="BD 1 Frequency 2", y=w1091) -> (x+y=w1090:u64)
                "BD1 Frequency Out 2" <- w1090
              }
              frame 3 {
                # "Fluorescence period"
              }
            }
            n583 = feedback-in #51(w806) -> ()
            n584 = feedback #51(w806) -> (w805:u32)
            n585 = Select(t=w808, s="Interlace ON/OFF", f="Interlace Off Parameters") -> (s? t:f=w846:u8)
            n586 = Subtract(x=w806, y=w805) -> (x-y=w804:u32)
            n587 = Subtract "The error"(x=w804, y=w803) -> (x-y=w781:u32)
            n588 = case shown="1, Default" w846 {
              tunnel: ["DIO count 1 (ticks)" "DIO count 2 (ticks)" "DIO count 3 (ticks)"] -> w802
              frame 1, Default {
              }
              frame 2 {
              }
              frame 3 {
              }
            }
            n589 = Number To Boolean Array(number=w781) -> (Boolean array=w782:bool[])
            n590 = Or Array Elements(Boolean array=w782) -> (logical OR=w780:bool)
            "DIO Late?" <- w780
            n591 = Boolean To (0,1)(Boolean=w780) -> (0, 1=w787:i16)
            n592 = To Unsigned Word Integer(number=w787) -> (unsigned 16bit integer=w784:u16)
            n593 = feedback #52(u16 0) -> (w785:u16)
            n594 = Add(x=w784, y=w785) -> (x+y=w783:u16)
            "DIO Late Counter" <- w783
            n595 = feedback-in #52(w783) -> ()
            n596 = Subtract(x=w802, y=w781) -> (x-y=w801:u32)
            n597 = Split Number(x=w843) -> (hi(x)=w842:u32, lo(x)=w841:u32)
            n598 = Split Number(x=w832) -> (hi(x)=w837:u32, lo(x)=w836:u32)
            n599 = Boolean To (0,1)(Boolean="+ phase (DIO)") -> (0, 1=w798:i16)
            n600 = Split Number(x=w842) -> (lo(x)=w840:u16)  [unwired: 1 out]
            n601 = Split Number(x=w841) -> (hi(x)=w839:u16, lo(x)=w838:u16)
            n602 = Split Number(x=w837) -> (lo(x)=w835:u16)  [unwired: 1 out]
            n603 = Split Number(x=w836) -> (hi(x)=w834:u16, lo(x)=w833:u16)
            n604 = Split Number(x=w791) -> (hi(x)=w793:u8, lo(x)=w792:u8)
            n605 = Split Number(x=w788) -> (hi(x)=w790:u8, lo(x)=w789:u8)
            n606 = Split Number(x=w840) -> (hi(x)=w830:u8, lo(x)=w829:u8)
            n607 = Split Number(x=w839) -> (hi(x)=w828:u8, lo(x)=w827:u8)
            n608 = Split Number(x=w835) -> (hi(x)=w823:u8, lo(x)=w822:u8)
            n609 = Split Number(x=w838) -> (hi(x)=w826:u8, lo(x)=w825:u8)
            n610 = Split Number(x=w834) -> (hi(x)=w821:u8, lo(x)=w820:u8)
            n611 = Split Number(x=w833) -> (hi(x)=w819:u8, lo(x)=w818:u8)
            n612 = Multiply(x=w798, y="Phase count adjustment (DIO)") -> (x*y=w794:i16)
            n613 = feedback #53(i16 0) -> (w796:i16)
            n614 = Subtract(x=w796, y=w794) -> (x-y=w795:i16)
            "DIO Relative phase" <- w795
            n615 = feedback-in #53(w795) -> ()
            n616 = Add(x=w801, y=w794) -> (x+y=w800:u32)
            n617 = Build Array "BD 1 A Stack"(w793, w792) -> (w815:u8[])
            n618 = Build Array "BD 2 A Stack"(w790, w789) -> (w814:u8[])
            n619 = Build Array "BD 1 nu Stack"(w830, w829, w828, w827, w826, w825) -> (w824:u8[])
            n620 = Build Array "BD 2 nu Stack"(w823, w822, w821, w820, w819, w818) -> (w817:u8[])
            n621 = case shown="2" w831 {
              tunnel: [w881 w884] -> w813
              tunnel: [u8 10 u8 4] -> w816
              tunnel: "Swap F1 and F2" -> [w882 w884]
              frame 2 {
                # "F2"
                n622 = Not(x=w882) -> (.not. x?=w881:bool)
              }
              frame 1, Default {
                # "low chooses F1"
                # "F1"
              }
            }
            n623 = case "If FPGA is controlling (toggling) RF synth" shown="True" w812 {
              tunnel: w824 -> [_ w860]
              tunnel: w817 -> [_ w859]
              tunnel: w816 -> [_ w858]
              tunnel: w815 -> [_ w857]
              tunnel: w814 -> [_ w856]
              frame False {
              }
              frame True {
                # "Write next amp.\n(wait until beginning of next loop iteration to update)"
                n624 = flat-sequence "Update the next F1 and F2 frequency value (the actual frequency won't change until FSK is switched).\nThen load the next amplitude value into buffer, but don't update it until the next cycle." {
                  tunnel: w860 -> [w863]
                  tunnel: w859 -> [w862]
                  tunnel: w858 -> [w861]
                  tunnel: w857 -> [w874]
                  tunnel: w856 -> [w873]
                  frame #0 {
                    n625 = for {
                      tunnel: w863 -> [w869] mode=indexing
                      tunnel: w862 -> [w868] mode=indexing
                      tunnel: w861 -> [w866]
                      i -> [w867]
                      # "Write next freq."
                      n626 = To Unsigned Byte Integer(number=w867) -> (unsigned 8bit integer=w864:u8)
                      n627 = Add(x=w866, y=w864) -> (x+y=w865:u8)
                      n628 = call "write to RF synth bd.vi"("Address Byte"=w865, "BD 2 Byte"=w868, "BD 1 Byte"=w869) -> ()
                    }
                  }
                  frame #1 {
                    # "send udclk high"
                    n629 = xnode "FPGA I/O Node"("Connector1/DIO30"=TRUE ("Connector1/DIO15")) -> ()  [unwired: 1 in, 1 out]
                  }
                  frame #2 {
                    n630 = xnode "FPGA I/O Node"("Connector1/DIO30"=FALSE ("Connector1/DIO15")) -> ()  [unwired: 1 in, 1 out]
                  }
                  frame #3 {
                    n631 = for {
                      tunnel: w874 -> [w880] mode=indexing
                      tunnel: w873 -> [w879] mode=indexing
                      tunnel: u8 33 -> [w877]
                      i -> [w878]
                      n632 = To Unsigned Byte Integer(number=w878) -> (unsigned 8bit integer=w875:u8)
                      n633 = Add(x=w877, y=w875) -> (x+y=w876:u8)
                      n634 = call "write to RF synth bd.vi"("Address Byte"=w876, "BD 2 Byte"=w879, "BD 1 Byte"=w880) -> ()
                    }
                  }
                }
              }
            }
          }
        }
      }
    }
  }
  n635 = node-c288(w5) -> ()
  n636 = while {
    shift-right: [w1125] -> _
    shift-left: w2 -> [w1127]
    tunnel: w3 -> [w1129]
    stop <- FALSE stop-if-true
    n637 = flat-sequence {
      tunnel: w1129 -> [_]
      tunnel: [w1130] -> w1128
      tunnel: w1127 -> [w1130]
      tunnel: w1128 -> [w1131]
      tunnel: [w1132] -> w1125
      frame #0 {
      }
      frame #1 {
        n638 = xnode "FPGA I/O Node"("Connector1/DIO32"=w1131, "Connector1/DIO33"=w1131, "Connector1/DIO34"=w1131) -> ()  [unwired: 3 in, 3 out]
      }
      frame #2 {
        n639 = case shown="0, Default" "Red operating mode" {
          tunnel: [TRUE FALSE FALSE] -> w1132
          frame 0, Default {
          }
          frame 1 {
          }
          frame 2 {
          }
        }
      }
    }
  }
